vi "Autonomous Independent.vi"() -> ()   [LabVIEW 2020]
doc: "This VI is called when autonomous begins, and will automatically be terminated when autonomous ends. You can carry out timed or sensor driven robot movement independently without needing to return to the caller."
uses:
  <vilib>/Rock Robotics/WPI/Solenoid/WPI_SolenoidValue.ctl
  <vilib>/Rock Robotics/WPI/Utilities/WPI_GetSetVariantRefNum.vi
  <vilib>/Rock Robotics/Network Tables/NT Read String.vi
  <vilib>/Rock Robotics/Network Tables/NT Write Numeric Array.vi
  <vilib>/Rock Robotics/WPI/Solenoid/WPI_SolenoidSetEnum.vi
  <vilib>/Rock Robotics/WPI/RobotDrive/WPI_RobotDriveArcadeDrive_Standard(NoSaturation).vi
  Robot Global Data.vi
panel:
  out "Current Movement, for debugging":T1 {"Y Joystick Value" scale=1.0..-1.0; "X Joystick Value" scale=-1.0..1.0}
  in  "Array of robot movements":T2(array[cluster])=[{"X Joystick Value"=0.39393939393939403, "Y Joystick Value"=0.0, "Delay (sec)"=1.0, "Movement Name"="turn"}, {"X Joystick Value"=-0.3737373737373737, "Y Joystick Value"=0.0, "Delay (sec)"=1.0, "Movement Name"="turn back"}] {"Y Joystick Value" scale=1.0..-1.0; "X Joystick Value" scale=-1.0..1.0}
  # "Be sure to right-click and choose Data Operations>>Make Current Value default if you want to save the array values with the VI"
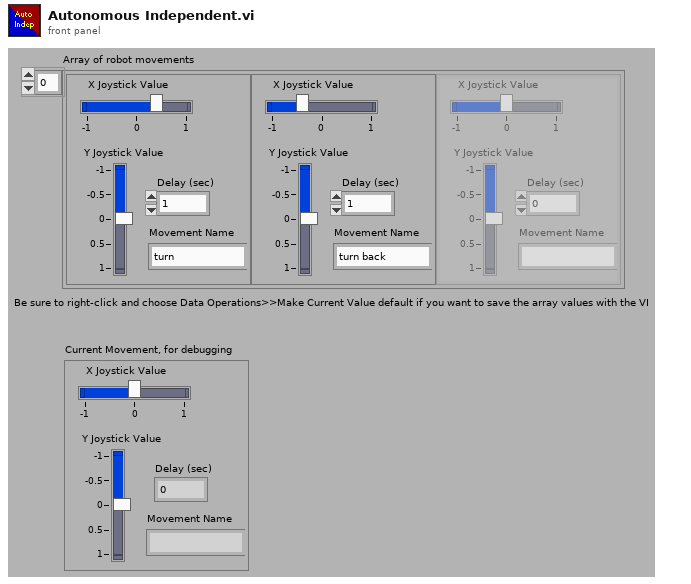
[diagram p1: front panel]
types:
  T1 = cluster{"X Joystick Value":dbl, "Y Joystick Value":dbl, "Delay (sec)":dbl, "Movement Name":string}
  T2 = cluster{"X Joystick Value":dbl, "Y Joystick Value":dbl, "Delay (sec)":dbl, "Movement Name":string}[]
  T3 = typedef "WPI_JoystickDevRef.ctl" = cluster{"Device":T4}
  T4 = typedef "WPI_JoystickDeviceEnum.ctl" = enum16{"USB 0", "USB 1", "USB 2", "USB 3", "USB 4", "USB 5"}
  T5 = typedef "WPI_SolenoidValue.ctl" = enum16{"Off", "On", "Forward", "Reverse"}
  T6 = typedef "WPI_MotorControlDeviceRef.ctl" = cluster{"DeviceStatus":errorcluster, "Type":T7, "PWM":cluster{"PWM Channel":T8, "DeadBand":T9}, "CAN":cluster{"Device Number":u8, "SetOutput VI Ref":variant, "GetOutput VI Ref":variant, "Enable VI Ref":variant, "Disable VI Ref":variant, "Data":variant}, "Invert":bool, "DIO PWM":cluster{"PWM \"Enable\" Channel":T8, "DIOChannel":T10, "PWM Rate":dbl}}
  T7 = typedef "WPI_MotorControlType.ctl" = enum16{"PWM", "CAN", "DIO PWM"}
  T8 = typedef "FPGA_DIOPWMChannel.ctl" = enum8{"PWM 0", "PWM 1", "PWM 2", "PWM 3", "PWM 4", "PWM 5", "PWM 6", "PWM 7", "PWM 8", "PWM 9", "PWM MXP 0", "PWM MXP 1", "PWM MXP 2", "PWM MXP 3", "PWM MXP 4", "PWM MXP 5", "PWM MXP 6", "PWM MXP 7", "PWM MXP 8", "PWM MXP 9", "Invalid"}
  T9 = typedef "WPI_PWMDeadband.ctl" = cluster{"Name":string, "maxPositivePwm":i32, "minPositivePwm":i32, "centerPwm":i32, "maxNegativePwm":i32, "minNegativePwm":i32, "angularRange":u16}
  T10 = typedef "FPGA_DIOChannel.ctl" = enum8{"DIO 0", "DIO 1", "DIO 2", "DIO 3", "DIO 4", "DIO 5", "DIO 6", "DIO 7", "DIO 8", "DIO 9", "DIO MXP 0", "DIO MXP 1", "DIO MXP 2", "DIO MXP 3", "DIO MXP 4", "DIO MXP 5", "DIO MXP 6", "DIO MXP 7", "DIO MXP 8", "DIO MXP 9", "DIO MXP 10", "DIO MXP 11", "DIO MXP 12", "DIO MXP 13", "DIO MXP 14", "DIO MXP 15", "SPI Port CS1", "SPI Port CS2", "SPI Port CS3", "SPI Port MISO", "SPI Port MOSI", "Invalid"}
  T11 = typedef "WPI_SolenoidDevRef.ctl" = cluster{"DevStatus":errorcluster, "Pneumatics Control Module":u8, "Forward Solenoid Channel":T12, "Reverse Solenoid Channel":T12}
  T12 = typedef "WPI_SolenoidChannel.ctl" = enum8{"Solenoid 0", "Solenoid 1", "Solenoid 2", "Solenoid 3", "Solenoid 4", "Solenoid 5", "Solenoid 6", "Solenoid 7", "Solenoid 8", "Solenoid 9", "Solenoid 10", "Solenoid 11", "Solenoid 12", "Solenoid 13", "Solenoid 14", "Solenoid 15", "Invalid"}
  T13 = typedef "WPI_RobotDriveDevRef.ctl" = cluster{"DevStatus":errorcluster, "Motors[]":T6[], "Square Inputs":bool, "Max Output":dbl}
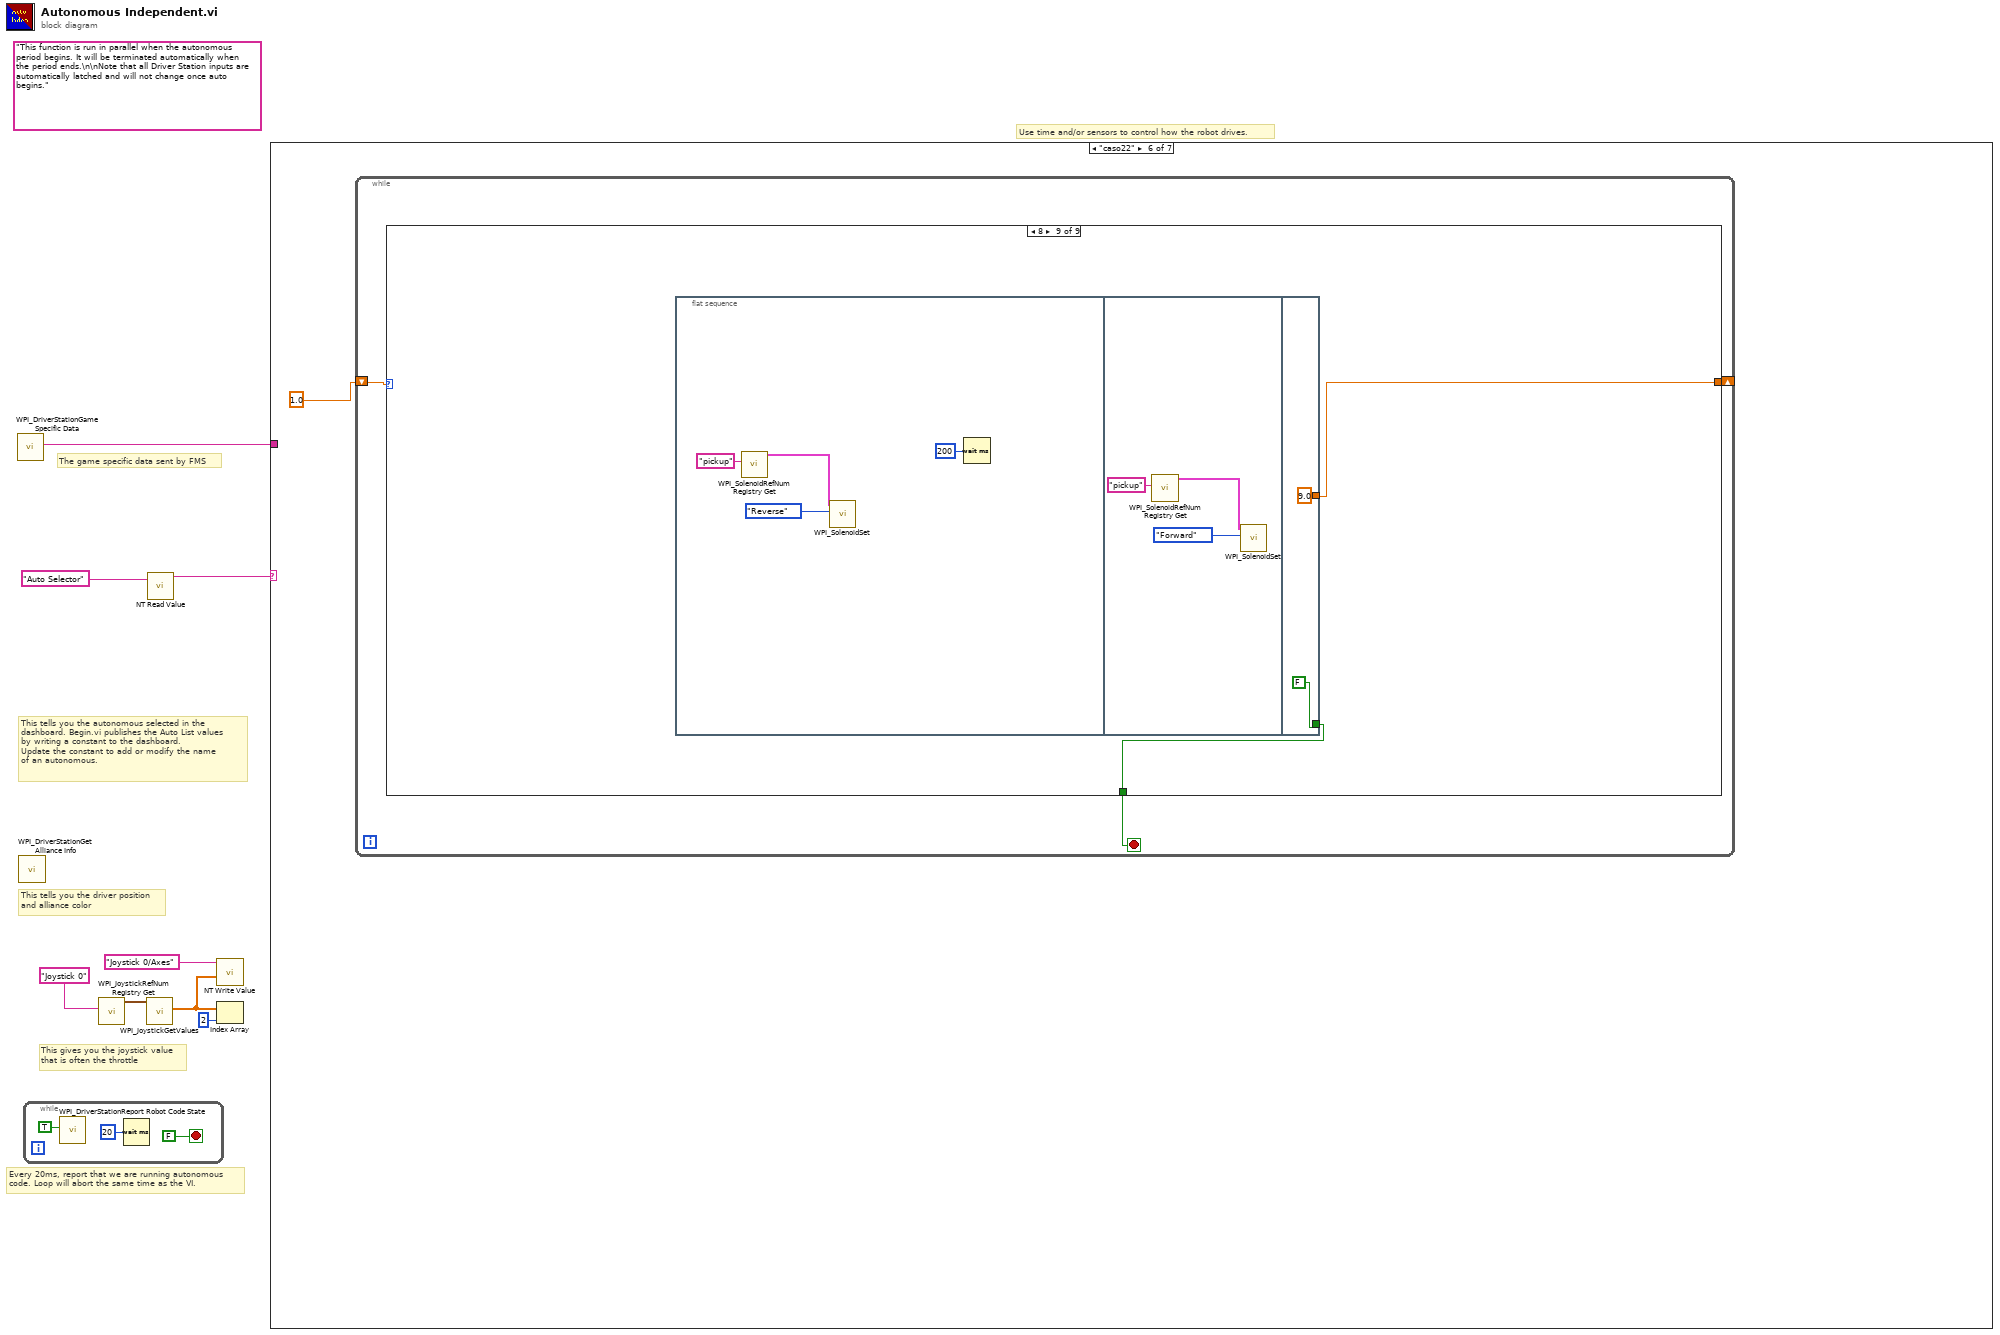
[diagram p0: block diagram]
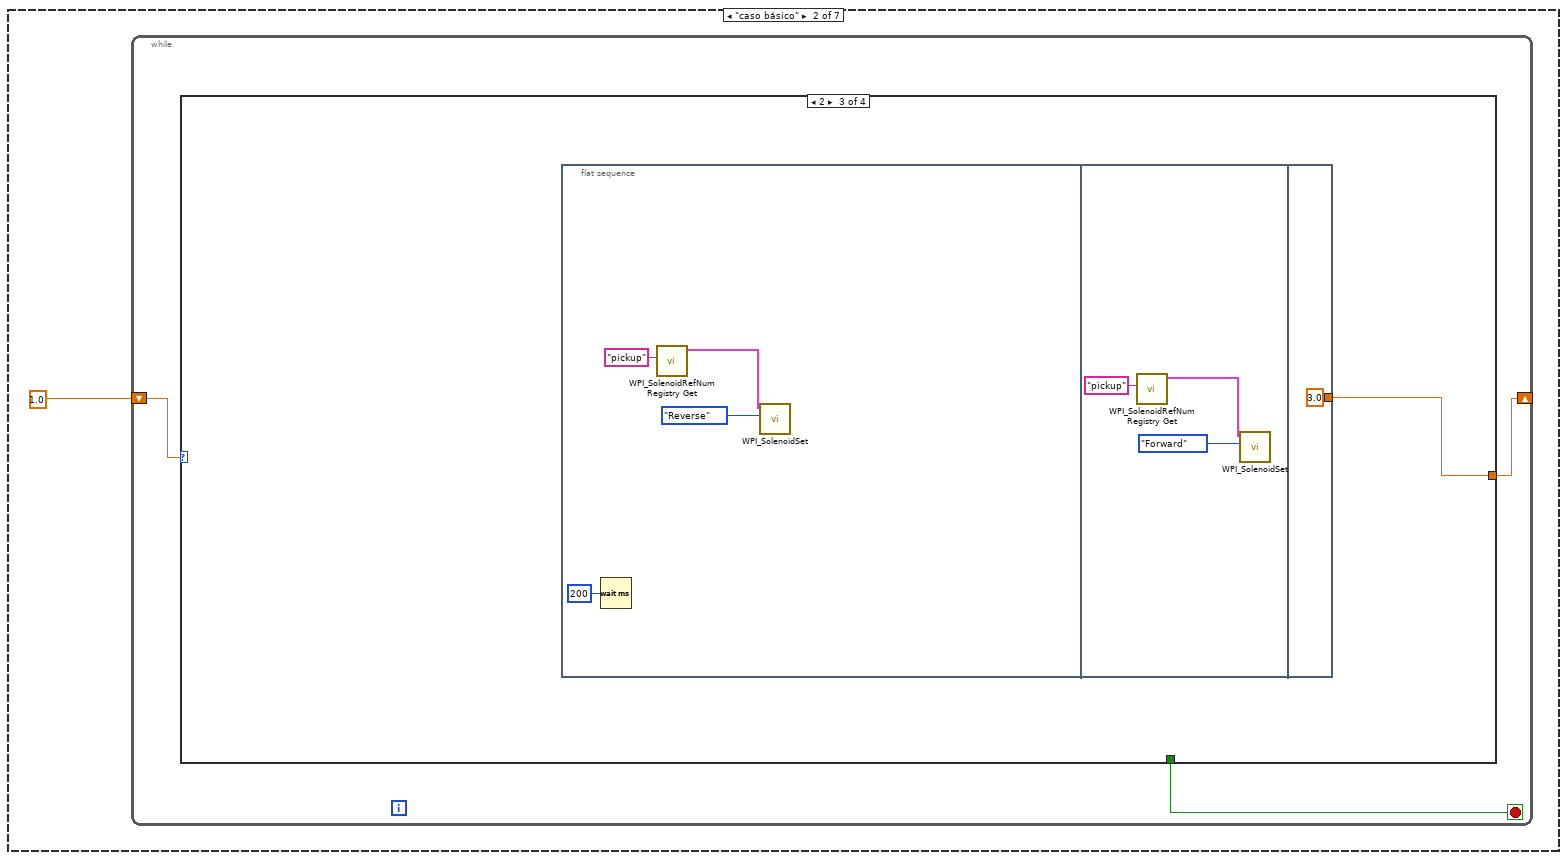
[diagram p3: hidden frame]
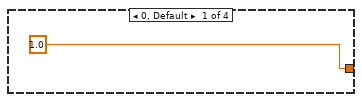
[diagram p4: hidden frame]
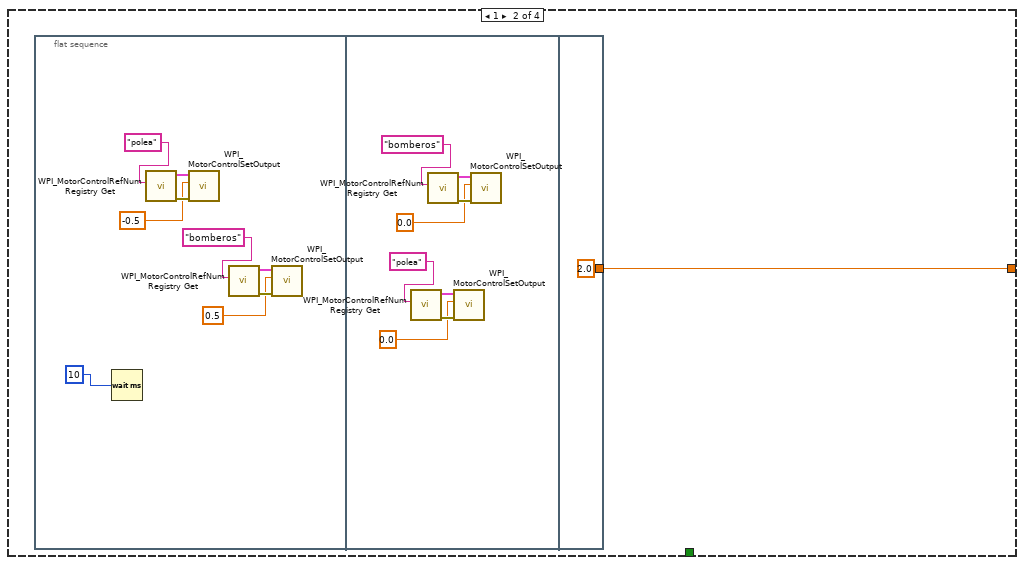
[diagram p5: hidden frame]
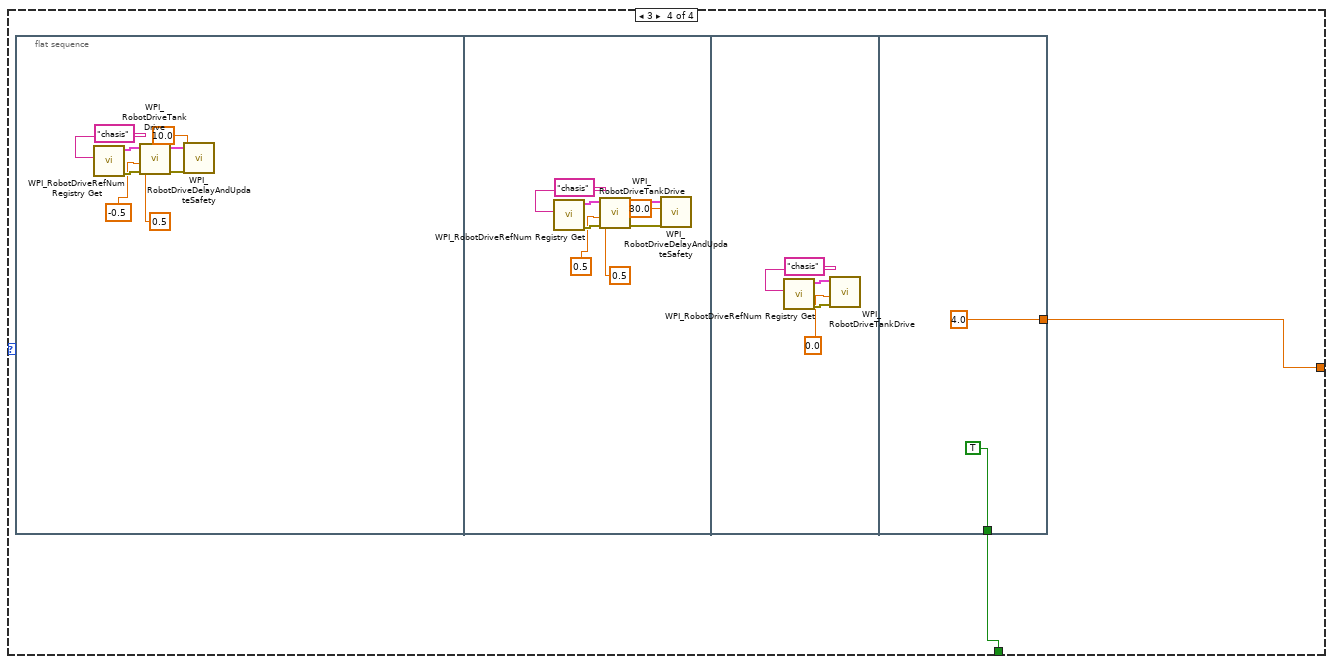
[diagram p6: hidden frame]
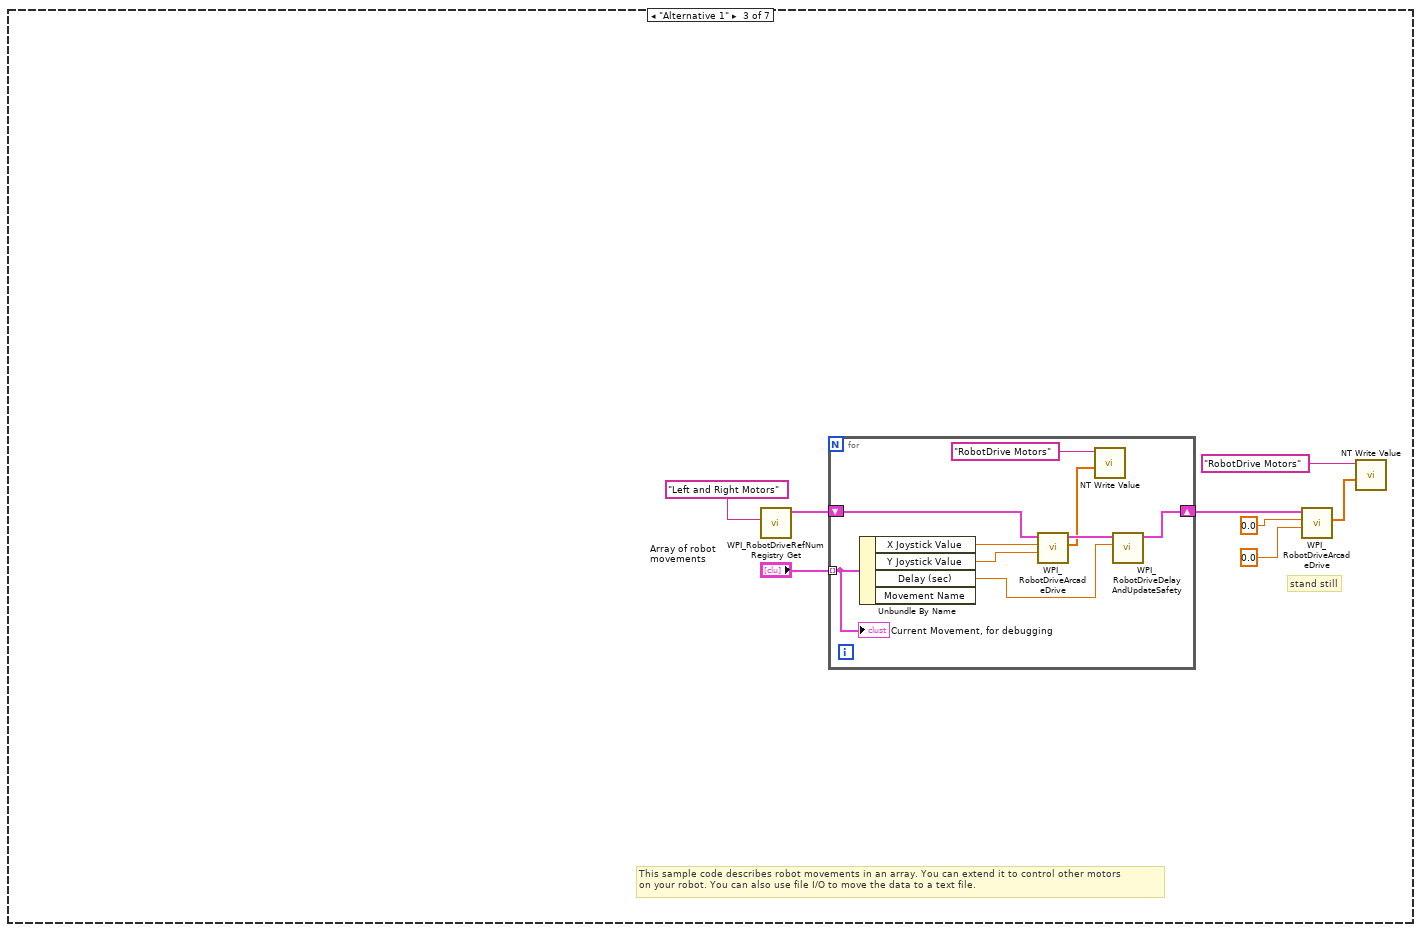
[diagram p7: hidden frame]
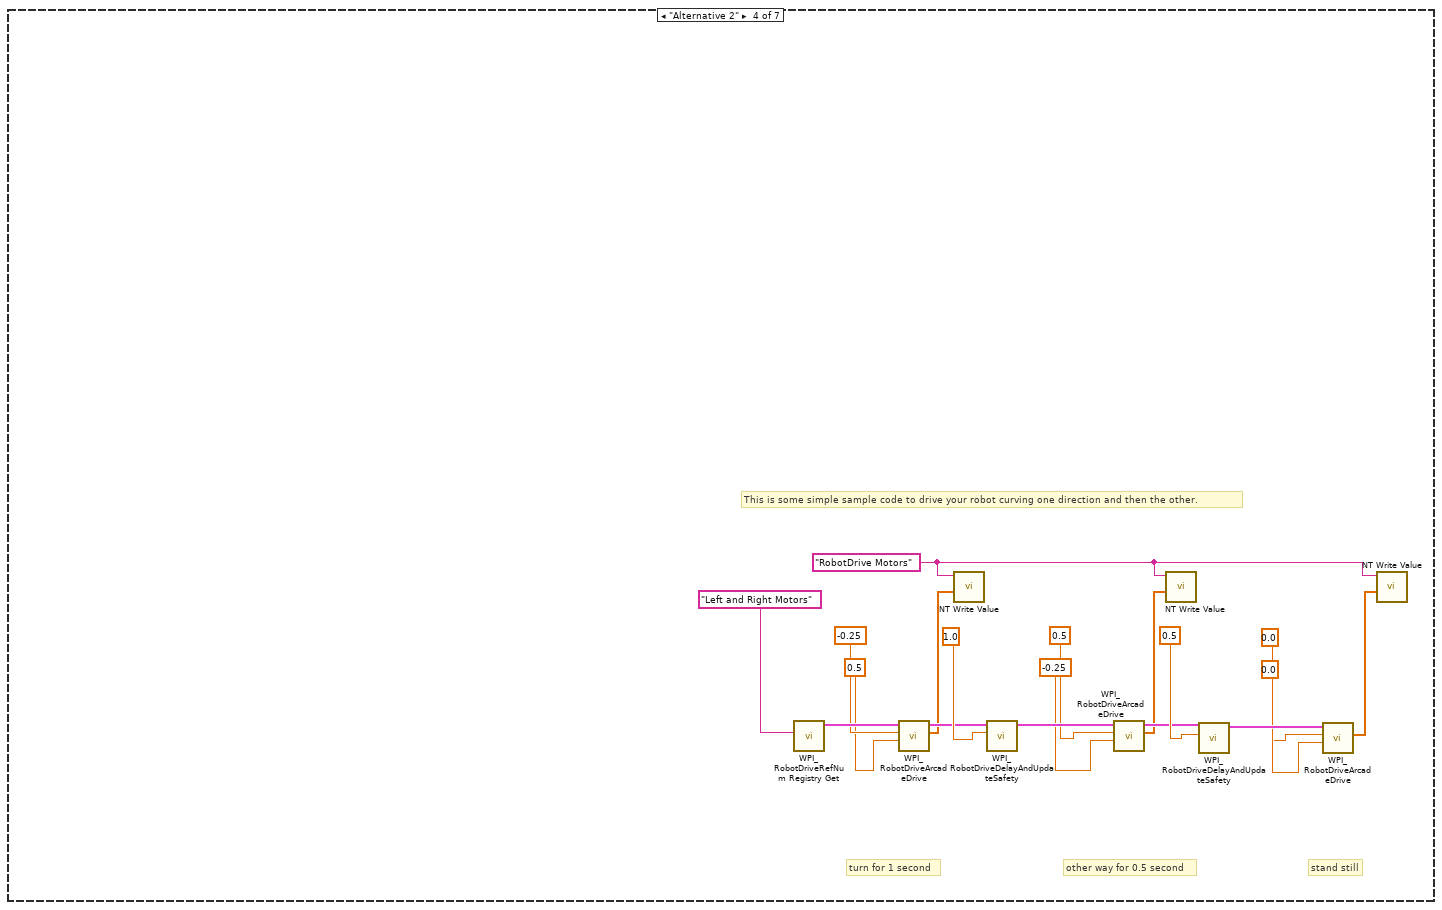
[diagram p8: hidden frame]
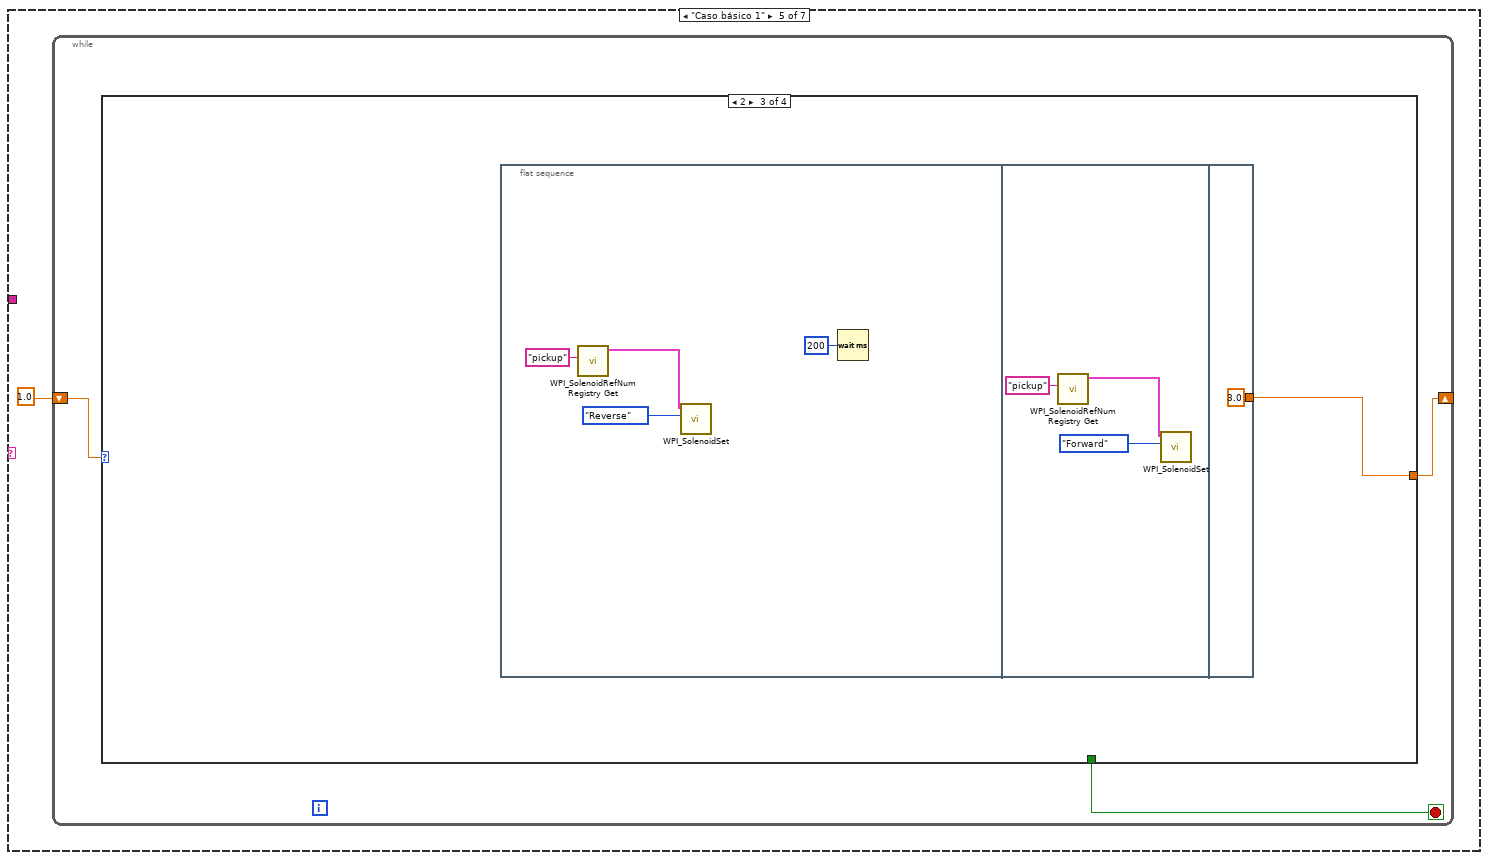
[diagram p9: hidden frame]
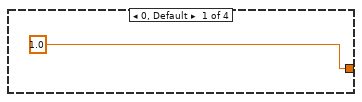
[diagram p10: hidden frame]
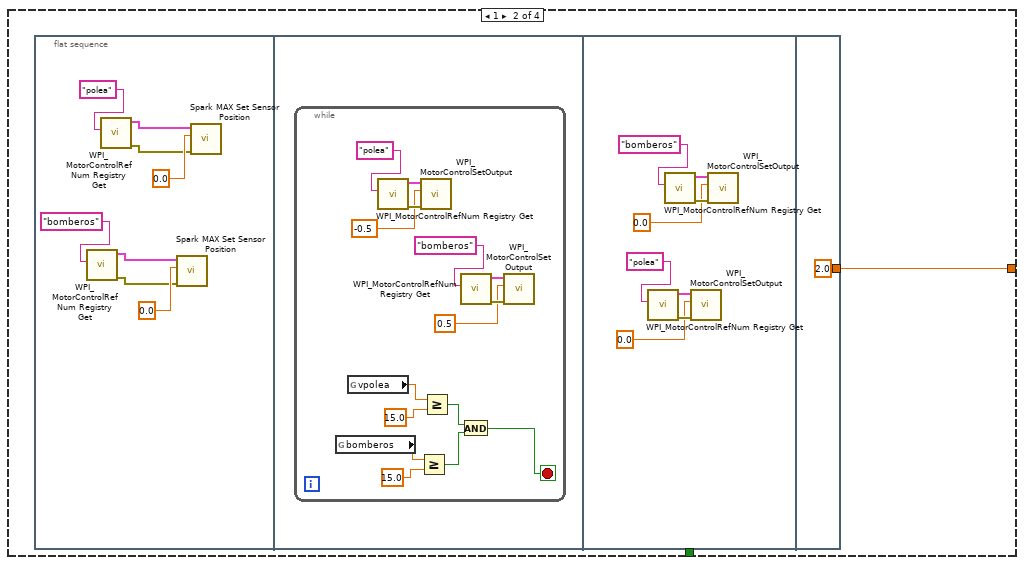
[diagram p11: hidden frame]
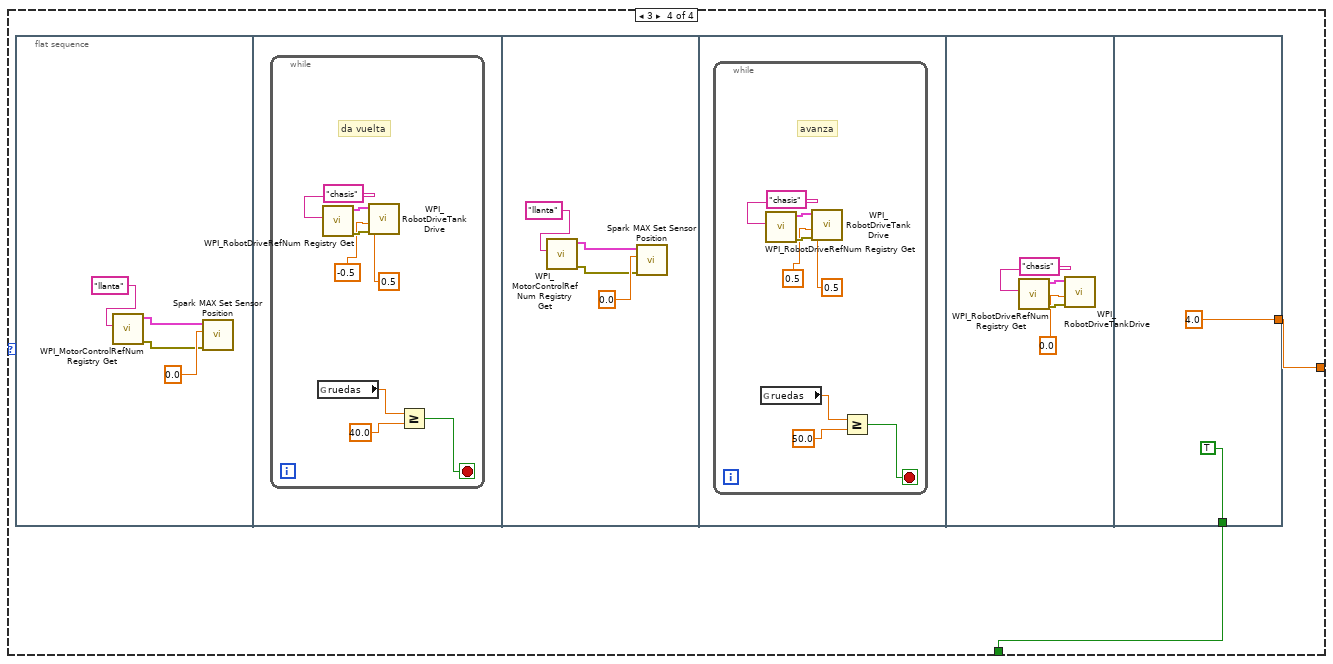
[diagram p12: hidden frame]
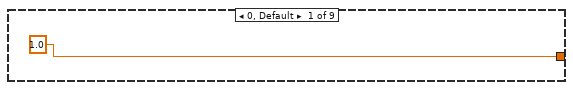
[diagram p13: hidden frame]
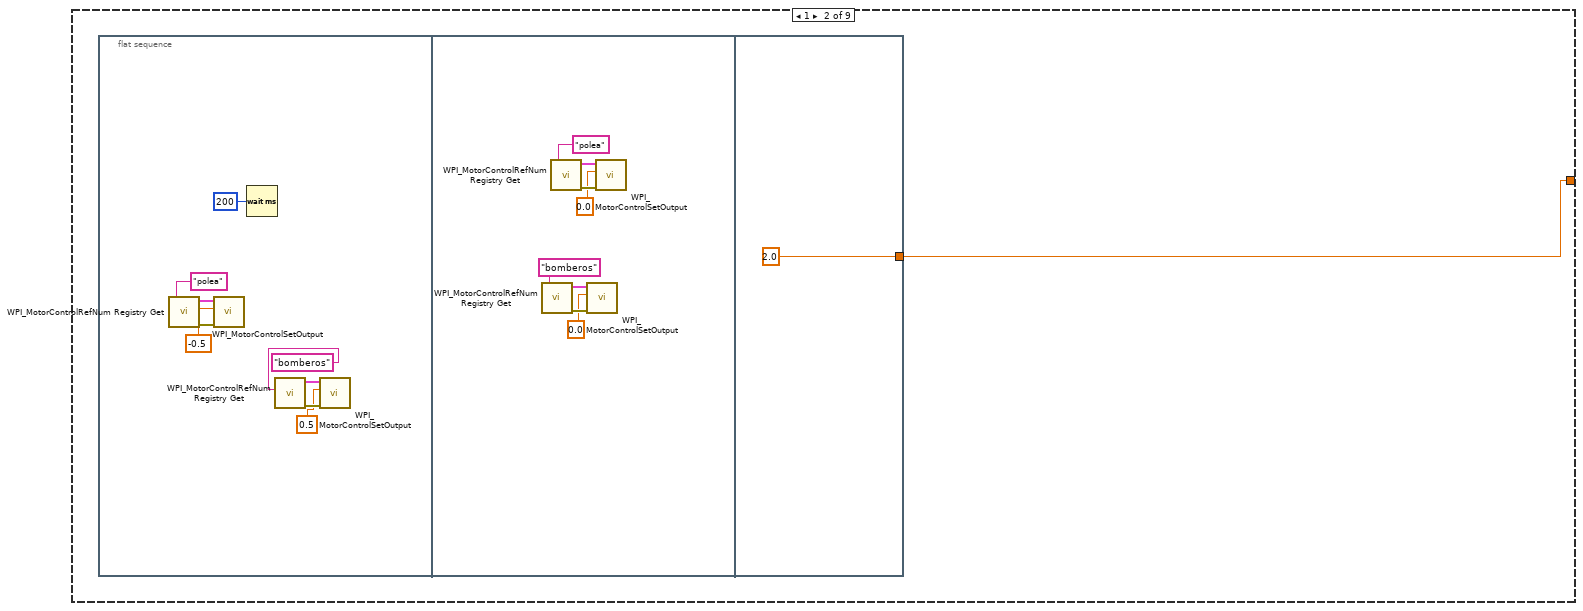
[diagram p14: hidden frame]
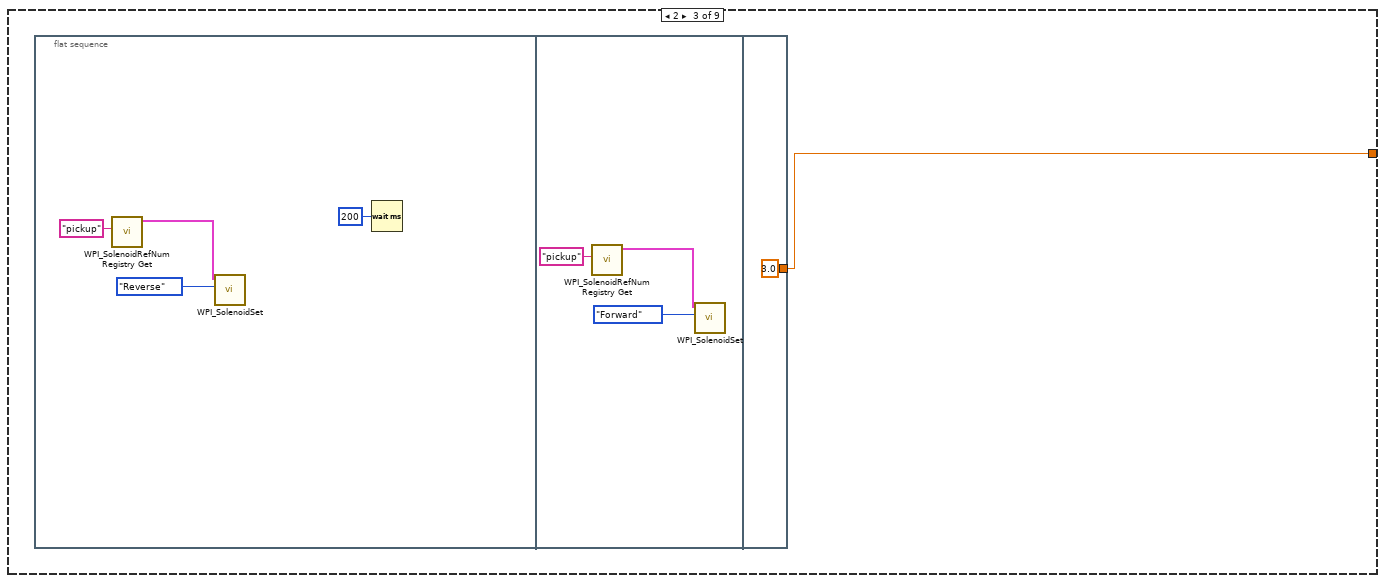
[diagram p15: hidden frame]
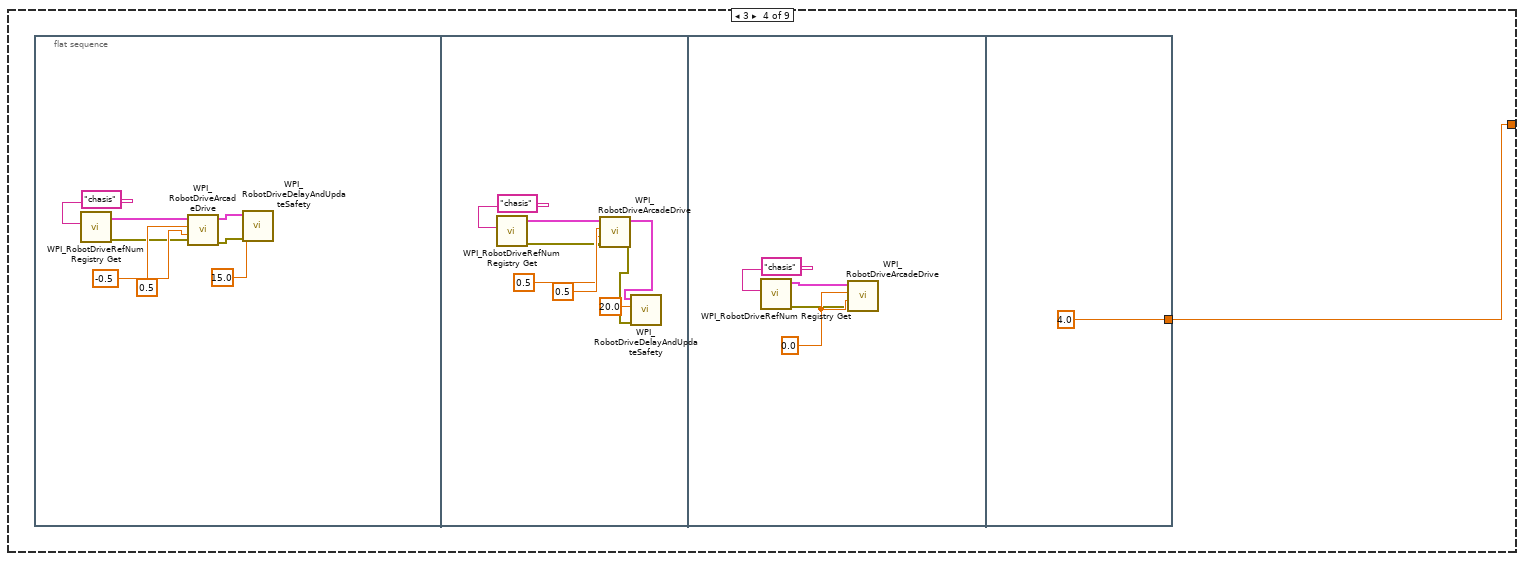
[diagram p16: hidden frame]
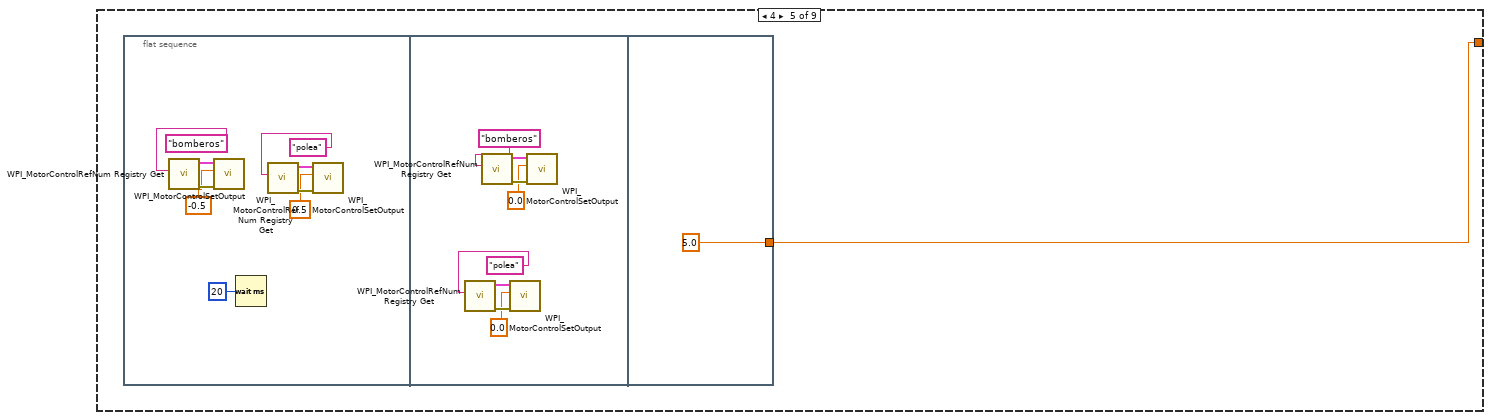
[diagram p17: hidden frame]
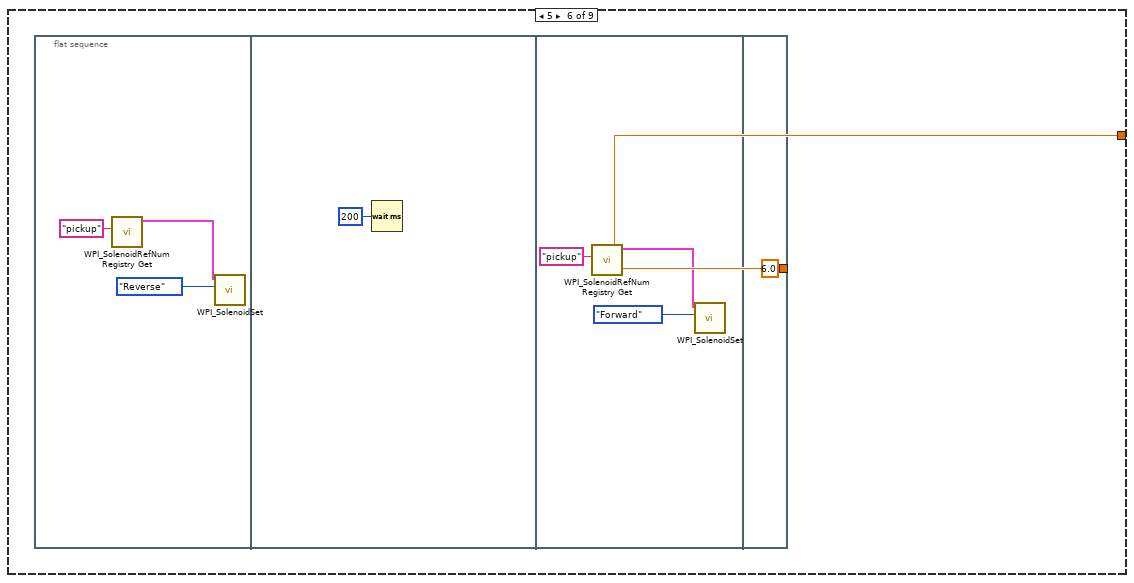
[diagram p18: hidden frame]
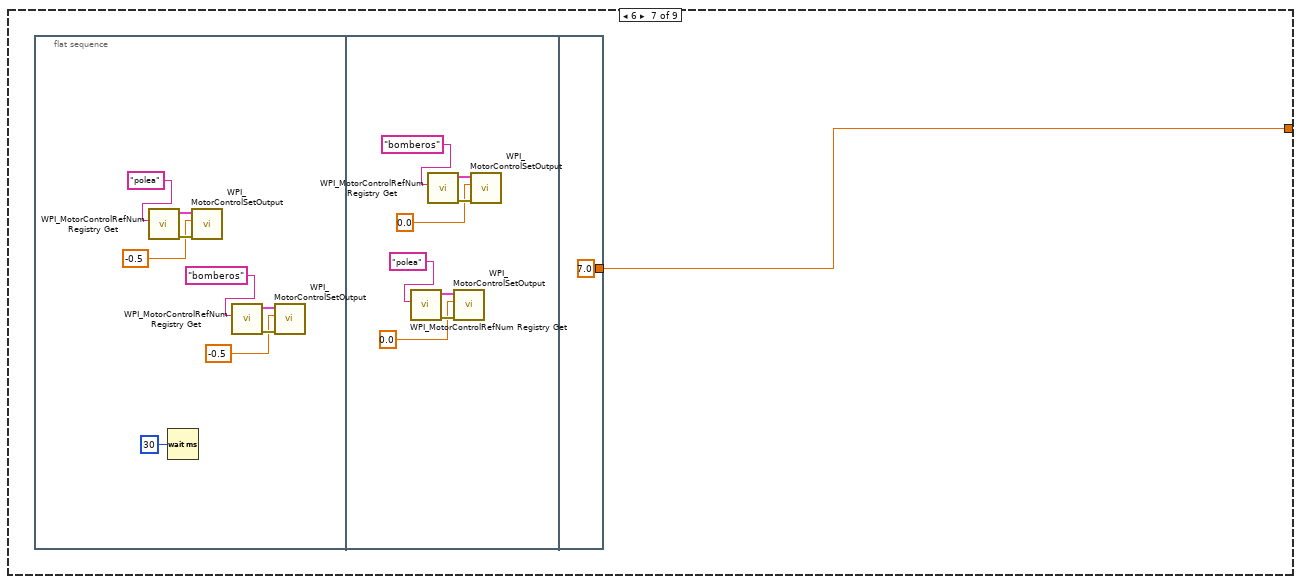
[diagram p19: hidden frame]
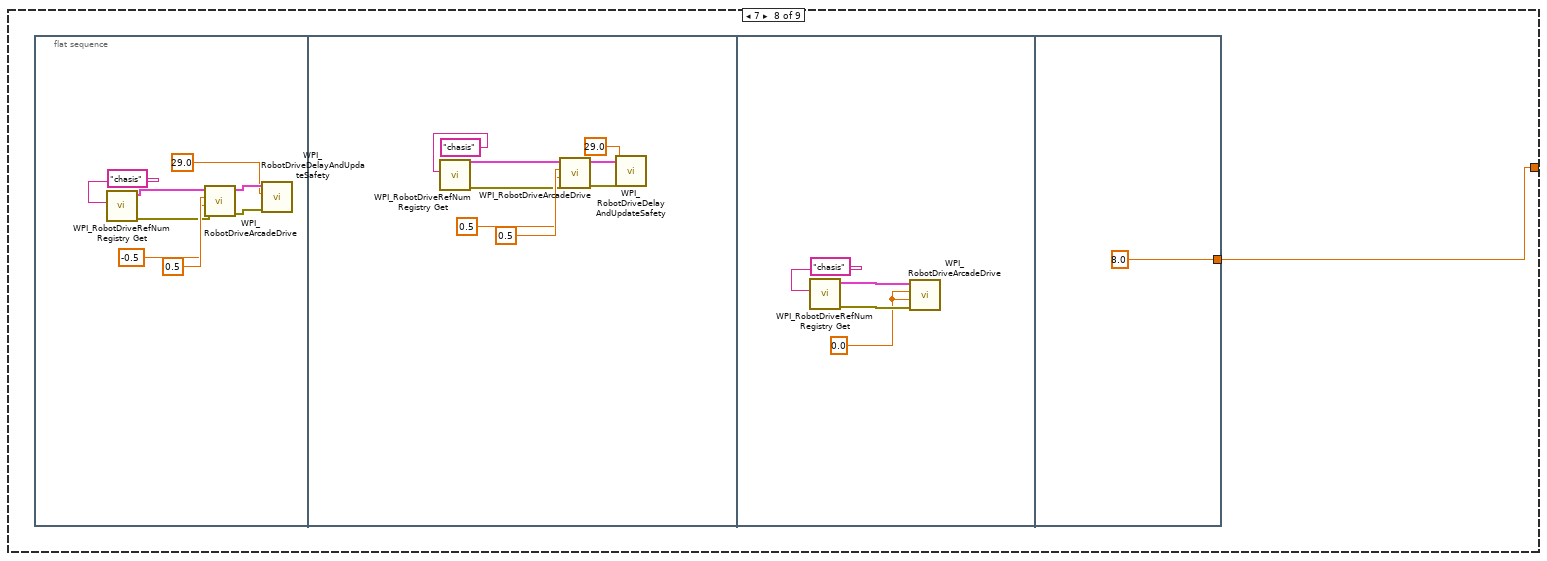
[diagram p20: hidden frame]
diagram:
  (unwired) "This function is run in parallel when the autonomous period begins. It will be terminated automatically when the period ends.\n\nNote that all Driver Station inputs are automatically latched and will not change once auto begins."
  # "The game specific data sent by FMS"
  # "This tells you the autonomous selected in the \ndashboard. Begin.vi publishes the Auto List values\nby writing a constant to the dashboard.\nUpdate the constant to add or modify the name\nof an autonomous."
  # "Every 20ms, report that we are running autonomous\ncode. Loop will abort the same time as the VI."
  # "This gives you the joystick value\nthat is often the throttle"
  # "Use time and/or sensors to control how the robot drives."
  # "This tells you the driver position\nand alliance color"
  n1 = call <vilib>:"WPI_DriverStationGame Specific Data.vi"() -> ("Game Specific Data"=w1:string)  [unwired: 11 in]
  n2 = call <vilib>:"WPI_DriverStationGet Alliance Info.vi"() -> ()  [unwired: 12 out]
  n3 = while {
    stop <- FALSE stop-if-true
    n4 = call <vilib>:"WPI_DriverStationReport Robot Code State.vi"("Autonomous"=TRUE) -> ()  [unwired: 10 in, 1 out]
    n5 = Wait (ms)(milliseconds to wait=u32 20) -> ()  [unwired: 1 out]
  }
  n6 = call <vilib>:"WPI_JoystickRefNum Registry Get.vi"("refnum name"="Joystick 0") -> ("JoystickDevRef"=w7:T3)  [unwired: 1 in, 9 out]
  n7 = call <vilib>:"WPI_JoystickGetValues.vi"("JoystickDevRef"=w7) -> ("Axes"=w3:dbl[])  [unwired: 6 in, 4 out]
  n8 = call-poly <vilib>:"NT Read Value.vi"("Name"="Auto Selector") -> ("String"=w4:string)  [unwired: 9 in, 1 out]
  n9 = call-poly <vilib>:"NT Write Value.vi"("Numeric Array"=w3, "Name"="Joystick 0/Axes") -> ()  [unwired: 9 in, 1 out]
  n10 = Index Array(array=w3, index=2) -> ()  [unwired: 1 out]
  n11 = case shown="\"caso22\"" w4 {
    tunnel: w1 -> [_ _ _ _ _ _ _]
    frame Default {
      # "You can put your main auto here, or you can right-click on the case and make any\nother frame be the default case."
      # "This is the frame that will execute if no selection is made, or if it is not recognized"
    }
    frame "caso básico" {
      n12 = while {
        shift-right: [w15] -> _
        shift-left: 1.0 -> [w13]
        stop <- w14 stop-if-true
        n13 = case shown="2" w13 {
          tunnel: [1.0 w17 w36 w46] -> w15
          tunnel: [_ _ _ w45] -> w14
          frame 0, Default {
          }
          frame 1 {
            n14 = flat-sequence {
              tunnel: [2.0] -> w17
              frame #0 {
                n15 = Wait (ms)(milliseconds to wait=u32 10 ("millisecond timer value")) -> ()  [unwired: 1 out]
                n16 = call <vilib>:"WPI_MotorControlRefNum Registry Get.vi"("refnum name"="polea") -> ("error out"=w26:errorcluster, "MotorControlDevRef"=w25:T6)  [unwired: 9 in]
                n17 = call <vilib>:"WPI_MotorControlSetOutput.vi"("error in (no error)"=w26, "Output"=-0.5, "MotorControlDevRef"=w25) -> ()  [unwired: 6 in, 3 out]
                n18 = call <vilib>:"WPI_MotorControlRefNum Registry Get.vi"("refnum name"="bomberos") -> ("error out"=w22:errorcluster, "MotorControlDevRef"=w21:T6)  [unwired: 9 in]
                n19 = call <vilib>:"WPI_MotorControlSetOutput.vi"("error in (no error)"=w22, "Output"=0.5, "MotorControlDevRef"=w21) -> ()  [unwired: 6 in, 3 out]
              }
              frame #1 {
                n20 = call <vilib>:"WPI_MotorControlRefNum Registry Get.vi"("refnum name"="polea") -> ("error out"=w33:errorcluster, "MotorControlDevRef"=w34:T6)  [unwired: 9 in]
                n21 = call <vilib>:"WPI_MotorControlRefNum Registry Get.vi"("refnum name"="bomberos") -> ("error out"=w29:errorcluster, "MotorControlDevRef"=w30:T6)  [unwired: 9 in]
                n22 = call <vilib>:"WPI_MotorControlSetOutput.vi"("error in (no error)"=w33, "Output"=0.0, "MotorControlDevRef"=w34) -> ()  [unwired: 6 in, 3 out]
                n23 = call <vilib>:"WPI_MotorControlSetOutput.vi"("error in (no error)"=w29, "Output"=0.0, "MotorControlDevRef"=w30) -> ()  [unwired: 6 in, 3 out]
              }
              frame #2 {
              }
            }
          }
          frame 2 {
            n24 = flat-sequence {
              tunnel: [3.0] -> w36
              frame #0 {
                n25 = Wait (ms)(milliseconds to wait=u32 200) -> ()  [unwired: 1 out]
                n26 = call <vilib>:"WPI_SolenoidRefNum Registry Get.vi"("refnum name"="pickup") -> ("SolenoidDevRef"=w40:T11)  [unwired: 9 in, 1 out]
                n27 = call-poly <vilib>:"WPI_SolenoidSet.vi"("Value"=WPI_SolenoidValue."Reverse", "SolenoidDevRef"=w40) -> ()  [unwired: 8 in, 2 out]
              }
              frame #1 {
                n28 = call <vilib>:"WPI_SolenoidRefNum Registry Get.vi"("refnum name"="pickup") -> ("SolenoidDevRef"=w43:T11)  [unwired: 9 in, 1 out]
                n29 = call-poly <vilib>:"WPI_SolenoidSet.vi"("Value"=WPI_SolenoidValue."Forward", "SolenoidDevRef"=w43) -> ()  [unwired: 8 in, 2 out]
              }
              frame #2 {
              }
            }
          }
          frame 3 {
            n30 = flat-sequence {
              tunnel: [4.0] -> w46
              tunnel: [TRUE] -> w45
              frame #0 {
                n31 = call <vilib>:"WPI_RobotDriveRefNum Registry Get.vi"("refnum name"="chasis") -> ("error out"=w54:errorcluster, "RobotDriveDevRef"=w53:T13)  [unwired: 9 in]
                n32 = call <vilib>:"WPI_RobotDriveTankDrive.vi"("error in (no error)"=w54, "Right axis value"=-0.5 ("Motor Output"), "Left axis value"=0.5 ("Motor Output"), "RobotDriveDevRef"=w53) -> ("error out"=w49:errorcluster, "RobotDriveDevRef"=w48:T13)  [unwired: 5 in, 1 out]
                n33 = call <vilib>:"WPI_RobotDriveDelayAndUpdateSafety.vi"("error in (no error)"=w49, "Delay (s)"=10.0, "RobotDriveDevRef"=w48) -> ()  [unwired: 7 in, 2 out]
              }
              frame #1 {
                n34 = call <vilib>:"WPI_RobotDriveRefNum Registry Get.vi"("refnum name"="chasis") -> ("error out"=w62:errorcluster, "RobotDriveDevRef"=w61:T13)  [unwired: 9 in]
                n35 = call <vilib>:"WPI_RobotDriveTankDrive.vi"("error in (no error)"=w62, "Right axis value"=0.5 ("Motor Output"), "Left axis value"=0.5 ("Motor Output"), "RobotDriveDevRef"=w61) -> ("error out"=w56:errorcluster, "RobotDriveDevRef"=w57:T13)  [unwired: 5 in, 1 out]
                n36 = call <vilib>:"WPI_RobotDriveDelayAndUpdateSafety.vi"("error in (no error)"=w56, "Delay (s)"=30.0, "RobotDriveDevRef"=w57) -> ()  [unwired: 7 in, 2 out]
              }
              frame #2 {
                n37 = call <vilib>:"WPI_RobotDriveRefNum Registry Get.vi"("refnum name"="chasis") -> ("error out"=w66:errorcluster, "RobotDriveDevRef"=w65:T13)  [unwired: 9 in]
                n38 = call <vilib>:"WPI_RobotDriveTankDrive.vi"("error in (no error)"=w66, "Right axis value"=0.0 ("Motor Output"), "RobotDriveDevRef"=w65) -> ()  [unwired: 6 in, 3 out]
              }
              frame #3 {
              }
            }
          }
        }
      }
    }
    frame "Alternative 1" {
      # "stand still"
      # "This sample code describes robot movements in an array. You can extend it to control other motors\non your robot. You can also use file I/O to move the data to a text file."
      n39 = call <vilib>:"WPI_RobotDriveRefNum Registry Get.vi"("refnum name"="Left and Right Motors") -> ("RobotDriveDevRef"=w75:T13)  [unwired: 1 in, 9 out]
      n40 = for {
        shift-right: [w83] -> w70
        shift-left: w75 -> [w84]
        tunnel: "Array of robot movements" -> [w79] mode=indexing
        n41 = Unbundle By Name(w79) -> ("X Joystick Value"=w82:dbl, "Y Joystick Value"=w81:dbl, "Delay (sec)"=w80:dbl)  [unwired: 1 out]
        n42 = call-poly <vilib>:"WPI_RobotDriveArcadeDrive.vi"("Y axis value"=w81, "X axis value"=w82, "RobotDriveDevRef"=w84) -> ("Motor Values"=w77:dbl[], "RobotDriveDevRef"=w85:T13)  [unwired: 1 in, 6 out]
        n43 = call-poly <vilib>:"NT Write Value.vi"("Numeric Array"=w77, "Name"="RobotDrive Motors") -> ()  [unwired: 9 in, 1 out]
        n44 = call <vilib>:"WPI_RobotDriveDelayAndUpdateSafety.vi"("Delay (s)"=w80, "RobotDriveDevRef"=w85) -> ("RobotDriveDevRef 2"=w83:T13)  [unwired: 8 in, 1 out]
        "Current Movement, for debugging" <- w79
      }
      n45 = call-poly <vilib>:"WPI_RobotDriveArcadeDrive.vi"("Y axis value"=0.0 ("X axis value"), "X axis value"=0.0, "RobotDriveDevRef"=w70) -> ("Motor Values"=w73:dbl[])  [unwired: 1 in, 7 out]
      n46 = call-poly <vilib>:"NT Write Value.vi"("Numeric Array"=w73, "Name"="RobotDrive Motors") -> ()  [unwired: 9 in, 1 out]
    }
    frame "Alternative 2" {
      w87 = "RobotDrive Motors" ("Name")
      # "This is some simple sample code to drive your robot curving one direction and then the other."
      # "stand still"
      # "other way for 0.5 second"
      # "turn for 1 second"
      n47 = call <vilib>:"WPI_RobotDriveRefNum Registry Get.vi"("refnum name"="Left and Right Motors") -> ("RobotDriveDevRef"=w103:T13)  [unwired: 1 in, 9 out]
      n48 = call-poly <vilib>:"WPI_RobotDriveArcadeDrive.vi"("Y axis value"=0.5 ("X axis value"), "X axis value"=-0.25, "RobotDriveDevRef"=w103) -> ("Motor Values"=w86:dbl[], "RobotDriveDevRef"=w96:T13)  [unwired: 1 in, 6 out]
      n49 = call-poly <vilib>:"NT Write Value.vi"("Numeric Array"=w86, "Name"=w87) -> ()  [unwired: 9 in, 1 out]
      n50 = call <vilib>:"WPI_RobotDriveDelayAndUpdateSafety.vi"("Delay (s)"=1.0, "RobotDriveDevRef"=w96) -> ("RobotDriveDevRef 2"=w97:T13)  [unwired: 8 in, 1 out]
      n51 = call-poly <vilib>:"WPI_RobotDriveArcadeDrive.vi"("Y axis value"=-0.25 ("X axis value"), "X axis value"=0.5, "RobotDriveDevRef"=w97) -> ("Motor Values"=w88:dbl[], "RobotDriveDevRef"=w98:T13)  [unwired: 1 in, 6 out]
      n52 = call-poly <vilib>:"NT Write Value.vi"("Numeric Array"=w88, "Name"=w87) -> ()  [unwired: 9 in, 1 out]
      n53 = call <vilib>:"WPI_RobotDriveDelayAndUpdateSafety.vi"("Delay (s)"=0.5, "RobotDriveDevRef"=w98) -> ("RobotDriveDevRef 2"=w99:T13)  [unwired: 8 in, 1 out]
      n54 = call-poly <vilib>:"WPI_RobotDriveArcadeDrive.vi"("Y axis value"=0.0 ("X axis value"), "X axis value"=0.0, "RobotDriveDevRef"=w99) -> ("Motor Values"=w89:dbl[])  [unwired: 1 in, 7 out]
      n55 = call-poly <vilib>:"NT Write Value.vi"("Numeric Array"=w89, "Name"=w87) -> ()  [unwired: 9 in, 1 out]
    }
    frame "Caso básico 1" {
      n56 = while {
        shift-right: [w107] -> _
        shift-left: 1.0 -> [w105]
        stop <- w106 stop-if-true
        n57 = case shown="2" w105 {
          tunnel: [1.0 w109 w142 w152] -> w107
          tunnel: [_ _ _ w151] -> w106
          frame 0, Default {
          }
          frame 1 {
            n58 = flat-sequence {
              tunnel: [2.0] -> w109
              frame #0 {
                n59 = call <vilib>:"WPI_MotorControlRefNum Registry Get.vi"("refnum name"="bomberos") -> ("error out"=w110:errorcluster, "MotorControlDevRef"=w111:T6)  [unwired: 9 in]
                n60 = call <vilib>:"WPI_MotorControlRefNum Registry Get.vi"("refnum name"="polea") -> ("error out"=w114:errorcluster, "MotorControlDevRef"=w115:T6)  [unwired: 9 in]
                n61 = call <vilib>:"Spark MAX Set Sensor Position.vi"("error in"=w110, "Position"=0.0, "MotorControlDeviceRef"=w111) -> ()  [unwired: 7 in, 2 out]
                n62 = call <vilib>:"Spark MAX Set Sensor Position.vi"("error in"=w114, "Position"=0.0, "MotorControlDeviceRef"=w115) -> ()  [unwired: 7 in, 2 out]
              }
              frame #1 {
                n63 = while {
                  stop <- w121 stop-if-true
                  n64 = global read "Robot Global Data.vi" "bomberos"() -> (w120:dbl)
                  n65 = global read "Robot Global Data.vi" "vpolea"() -> (w128:dbl)
                  n66 = call <vilib>:"WPI_MotorControlRefNum Registry Get.vi"("refnum name"="polea") -> ("error out"=w132:errorcluster, "MotorControlDevRef"=w131:T6)  [unwired: 9 in]
                  n67 = Greater Or Equal?(x=w120, y=15.0) -> (x >= y?=w118:bool)
                  n68 = call <vilib>:"WPI_MotorControlSetOutput.vi"("error in (no error)"=w132, "Output"=-0.5, "MotorControlDevRef"=w131) -> ()  [unwired: 6 in, 3 out]
                  n69 = Greater Or Equal?(x=w128, y=15.0) -> (x >= y?=w122:bool)
                  n70 = call <vilib>:"WPI_MotorControlRefNum Registry Get.vi"("refnum name"="bomberos") -> ("error out"=w126:errorcluster, "MotorControlDevRef"=w125:T6)  [unwired: 9 in]
                  n71 = And(x=w122, y=w118) -> (x .and. y?=w121:bool)
                  n72 = call <vilib>:"WPI_MotorControlSetOutput.vi"("error in (no error)"=w126, "Output"=0.5, "MotorControlDevRef"=w125) -> ()  [unwired: 6 in, 3 out]
                }
              }
              frame #2 {
                n73 = call <vilib>:"WPI_MotorControlRefNum Registry Get.vi"("refnum name"="polea") -> ("error out"=w139:errorcluster, "MotorControlDevRef"=w140:T6)  [unwired: 9 in]
                n74 = call <vilib>:"WPI_MotorControlRefNum Registry Get.vi"("refnum name"="bomberos") -> ("error out"=w135:errorcluster, "MotorControlDevRef"=w136:T6)  [unwired: 9 in]
                n75 = call <vilib>:"WPI_MotorControlSetOutput.vi"("error in (no error)"=w139, "Output"=0.0, "MotorControlDevRef"=w140) -> ()  [unwired: 6 in, 3 out]
                n76 = call <vilib>:"WPI_MotorControlSetOutput.vi"("error in (no error)"=w135, "Output"=0.0, "MotorControlDevRef"=w136) -> ()  [unwired: 6 in, 3 out]
              }
              frame #3 {
              }
            }
          }
          frame 2 {
            n77 = flat-sequence {
              tunnel: [3.0] -> w142
              frame #0 {
                n78 = call <vilib>:"WPI_SolenoidRefNum Registry Get.vi"("refnum name"="pickup") -> ("SolenoidDevRef"=w145:T11)  [unwired: 9 in, 1 out]
                n79 = call-poly <vilib>:"WPI_SolenoidSet.vi"("Value"=WPI_SolenoidValue."Reverse", "SolenoidDevRef"=w145) -> ()  [unwired: 8 in, 2 out]
                n80 = Wait (ms)(milliseconds to wait=u32 200) -> ()  [unwired: 1 out]
              }
              frame #1 {
                n81 = call <vilib>:"WPI_SolenoidRefNum Registry Get.vi"("refnum name"="pickup") -> ("SolenoidDevRef"=w149:T11)  [unwired: 9 in, 1 out]
                n82 = call-poly <vilib>:"WPI_SolenoidSet.vi"("Value"=WPI_SolenoidValue."Forward", "SolenoidDevRef"=w149) -> ()  [unwired: 8 in, 2 out]
              }
              frame #2 {
              }
            }
          }
          frame 3 {
            n83 = flat-sequence {
              tunnel: [4.0] -> w152
              tunnel: [TRUE] -> w151
              frame #0 {
                n84 = call <vilib>:"WPI_MotorControlRefNum Registry Get.vi"("refnum name"="llanta") -> ("error out"=w153:errorcluster, "MotorControlDevRef"=w154:T6)  [unwired: 9 in]
                n85 = call <vilib>:"Spark MAX Set Sensor Position.vi"("error in"=w153, "Position"=0.0, "MotorControlDeviceRef"=w154) -> ()  [unwired: 7 in, 2 out]
              }
              frame #1 {
                n86 = while {
                  stop <- w157 stop-if-true
                  # "da vuelta"
                  n87 = global read "Robot Global Data.vi" "ruedas"() -> (w159:dbl)
                  n88 = call <vilib>:"WPI_RobotDriveRefNum Registry Get.vi"("refnum name"="chasis") -> ("error out"=w164:errorcluster, "RobotDriveDevRef"=w163:T13)  [unwired: 9 in]
                  n89 = call <vilib>:"WPI_RobotDriveTankDrive.vi"("error in (no error)"=w164, "Right axis value"=-0.5 ("Motor Output"), "Left axis value"=0.5 ("Motor Output"), "RobotDriveDevRef"=w163) -> ()  [unwired: 5 in, 3 out]
                  n90 = Greater Or Equal?(x=w159, y=40.0) -> (x >= y?=w157:bool)
                }
              }
              frame #2 {
                n91 = call <vilib>:"WPI_MotorControlRefNum Registry Get.vi"("refnum name"="llanta") -> ("error out"=w165:errorcluster, "MotorControlDevRef"=w166:T6)  [unwired: 9 in]
                n92 = call <vilib>:"Spark MAX Set Sensor Position.vi"("error in"=w165, "Position"=0.0, "MotorControlDeviceRef"=w166) -> ()  [unwired: 7 in, 2 out]
              }
              frame #3 {
                n93 = while {
                  stop <- w169 stop-if-true
                  # "avanza"
                  n94 = global read "Robot Global Data.vi" "ruedas"() -> (w171:dbl)
                  n95 = call <vilib>:"WPI_RobotDriveRefNum Registry Get.vi"("refnum name"="chasis") -> ("error out"=w176:errorcluster, "RobotDriveDevRef"=w175:T13)  [unwired: 9 in]
                  n96 = call <vilib>:"WPI_RobotDriveTankDrive.vi"("error in (no error)"=w176, "Right axis value"=0.5 ("Motor Output"), "Left axis value"=0.5 ("Motor Output"), "RobotDriveDevRef"=w175) -> ()  [unwired: 5 in, 3 out]
                  n97 = Greater Or Equal?(x=w171, y=50.0) -> (x >= y?=w169:bool)
                }
              }
              frame #4 {
                n98 = call <vilib>:"WPI_RobotDriveRefNum Registry Get.vi"("refnum name"="chasis") -> ("error out"=w180:errorcluster, "RobotDriveDevRef"=w179:T13)  [unwired: 9 in]
                n99 = call <vilib>:"WPI_RobotDriveTankDrive.vi"("error in (no error)"=w180, "Right axis value"=0.0 ("Motor Output"), "RobotDriveDevRef"=w179) -> ()  [unwired: 6 in, 3 out]
              }
              frame #5 {
              }
            }
          }
        }
      }
    }
    frame "caso22" {
      n100 = while {
        shift-right: [w185] -> _
        shift-left: 1.0 -> [w186]
        stop <- w184 stop-if-true
        n101 = case shown="8" w186 {
          tunnel: [1.0 w188 w207 w216 w238 w257 w266 w285 w308] -> w185
          tunnel: [_ _ _ _ _ _ _ _ w307] -> w184
          frame 0, Default {
          }
          frame 1 {
            n102 = flat-sequence {
              tunnel: [2.0] -> w188
              frame #0 {
                n103 = call <vilib>:"WPI_MotorControlRefNum Registry Get.vi"("refnum name"="polea") -> ("error out"=w196:errorcluster, "MotorControlDevRef"=w197:T6)  [unwired: 9 in]
                n104 = call <vilib>:"WPI_MotorControlSetOutput.vi"("error in (no error)"=w196, "Output"=-0.5 ("Motor Output"), "MotorControlDevRef"=w197) -> ()  [unwired: 6 in, 3 out]
                n105 = Wait (ms)(milliseconds to wait=u32 200) -> ()  [unwired: 1 out]
                n106 = call <vilib>:"WPI_MotorControlRefNum Registry Get.vi"("refnum name"="bomberos") -> ("error out"=w193:errorcluster, "MotorControlDevRef"=w192:T6)  [unwired: 9 in]
                n107 = call <vilib>:"WPI_MotorControlSetOutput.vi"("error in (no error)"=w193, "Output"=0.5 ("Motor Output"), "MotorControlDevRef"=w192) -> ()  [unwired: 6 in, 3 out]
              }
              frame #1 {
                n108 = call <vilib>:"WPI_MotorControlRefNum Registry Get.vi"("refnum name"="bomberos") -> ("error out"=w200:errorcluster, "MotorControlDevRef"=w201:T6)  [unwired: 9 in]
                n109 = call <vilib>:"WPI_MotorControlRefNum Registry Get.vi"("refnum name"="polea") -> ("error out"=w204:errorcluster, "MotorControlDevRef"=w205:T6)  [unwired: 9 in]
                n110 = call <vilib>:"WPI_MotorControlSetOutput.vi"("error in (no error)"=w200, "Output"=0.0 ("Motor Output"), "MotorControlDevRef"=w201) -> ()  [unwired: 6 in, 3 out]
                n111 = call <vilib>:"WPI_MotorControlSetOutput.vi"("error in (no error)"=w204, "Output"=0.0 ("Motor Output"), "MotorControlDevRef"=w205) -> ()  [unwired: 6 in, 3 out]
              }
              frame #2 {
              }
            }
          }
          frame 2 {
            n112 = flat-sequence {
              tunnel: [3.0] -> w207
              frame #0 {
                n113 = call <vilib>:"WPI_SolenoidRefNum Registry Get.vi"("refnum name"="pickup") -> ("SolenoidDevRef"=w210:T11)  [unwired: 9 in, 1 out]
                n114 = call-poly <vilib>:"WPI_SolenoidSet.vi"("Value"=WPI_SolenoidValue."Reverse", "SolenoidDevRef"=w210) -> ()  [unwired: 8 in, 2 out]
                n115 = Wait (ms)(milliseconds to wait=u32 200) -> ()  [unwired: 1 out]
              }
              frame #1 {
                n116 = call <vilib>:"WPI_SolenoidRefNum Registry Get.vi"("refnum name"="pickup") -> ("SolenoidDevRef"=w214:T11)  [unwired: 9 in, 1 out]
                n117 = call-poly <vilib>:"WPI_SolenoidSet.vi"("Value"=WPI_SolenoidValue."Forward", "SolenoidDevRef"=w214) -> ()  [unwired: 8 in, 2 out]
              }
              frame #2 {
              }
            }
          }
          frame 3 {
            n118 = flat-sequence {
              tunnel: [4.0] -> w216
              frame #0 {
                n119 = call <vilib>:"WPI_RobotDriveRefNum Registry Get.vi"("refnum name"="chasis") -> ("error out"=w220:errorcluster, "RobotDriveDevRef"=w221:T13)  [unwired: 9 in]
                n120 = call-poly <vilib>:"WPI_RobotDriveArcadeDrive.vi"("error in (no error)"=w220, "Y axis value"=-0.5 ("Motor Output"), "X axis value"=0.5 ("Motor Output"), "RobotDriveDevRef"=w221) -> ("error out"=w219:errorcluster, "RobotDriveDevRef"=w218:T13)  [unwired: 5 in, 1 out]
                n121 = call <vilib>:"WPI_RobotDriveDelayAndUpdateSafety.vi"("error in (no error)"=w219, "Delay (s)"=15.0, "RobotDriveDevRef"=w218) -> ()  [unwired: 7 in, 2 out]
              }
              frame #1 {
                n122 = call <vilib>:"WPI_RobotDriveRefNum Registry Get.vi"("refnum name"="chasis") -> ("error out"=w228:errorcluster, "RobotDriveDevRef"=w229:T13)  [unwired: 9 in]
                n123 = call-poly <vilib>:"WPI_RobotDriveArcadeDrive.vi"("error in (no error)"=w228, "Y axis value"=0.5 ("Motor Output"), "X axis value"=0.5 ("Motor Output"), "RobotDriveDevRef"=w229) -> ("error out"=w226:errorcluster, "RobotDriveDevRef"=w227:T13)  [unwired: 5 in, 1 out]
                n124 = call <vilib>:"WPI_RobotDriveDelayAndUpdateSafety.vi"("error in (no error)"=w226, "Delay (s)"=20.0, "RobotDriveDevRef"=w227) -> ()  [unwired: 7 in, 2 out]
              }
              frame #2 {
                w235 = 0.0 ("Motor Output")
                n125 = call <vilib>:"WPI_RobotDriveRefNum Registry Get.vi"("refnum name"="chasis") -> ("error out"=w233:errorcluster, "RobotDriveDevRef"=w234:T13)  [unwired: 9 in]
                n126 = call-poly <vilib>:"WPI_RobotDriveArcadeDrive.vi"("error in (no error)"=w233, "Y axis value"=w235, "X axis value"=w235, "RobotDriveDevRef"=w234) -> ()  [unwired: 5 in, 3 out]
              }
              frame #3 {
              }
            }
          }
          frame 4 {
            n127 = flat-sequence {
              tunnel: [5.0] -> w238
              frame #0 {
                n128 = call <vilib>:"WPI_MotorControlRefNum Registry Get.vi"("refnum name"="bomberos") -> ("error out"=w247:errorcluster, "MotorControlDevRef"=w246:T6)  [unwired: 9 in]
                n129 = call <vilib>:"WPI_MotorControlSetOutput.vi"("error in (no error)"=w247, "Output"=-0.5 ("Motor Output"), "MotorControlDevRef"=w246) -> ()  [unwired: 6 in, 3 out]
                n130 = Wait (ms)(milliseconds to wait=u32 20) -> ()  [unwired: 1 out]
                n131 = call <vilib>:"WPI_MotorControlRefNum Registry Get.vi"("refnum name"="polea") -> ("error out"=w243:errorcluster, "MotorControlDevRef"=w242:T6)  [unwired: 9 in]
                n132 = call <vilib>:"WPI_MotorControlSetOutput.vi"("error in (no error)"=w243, "Output"=0.5 ("Motor Output"), "MotorControlDevRef"=w242) -> ()  [unwired: 6 in, 3 out]
              }
              frame #1 {
                n133 = call <vilib>:"WPI_MotorControlRefNum Registry Get.vi"("refnum name"="polea") -> ("error out"=w254:errorcluster, "MotorControlDevRef"=w255:T6)  [unwired: 9 in]
                n134 = call <vilib>:"WPI_MotorControlRefNum Registry Get.vi"("refnum name"="bomberos") -> ("error out"=w252:errorcluster, "MotorControlDevRef"=w253:T6)  [unwired: 9 in]
                n135 = call <vilib>:"WPI_MotorControlSetOutput.vi"("error in (no error)"=w254, "Output"=0.0 ("Motor Output"), "MotorControlDevRef"=w255) -> ()  [unwired: 6 in, 3 out]
                n136 = call <vilib>:"WPI_MotorControlSetOutput.vi"("error in (no error)"=w252, "Output"=0.0 ("Motor Output"), "MotorControlDevRef"=w253) -> ()  [unwired: 6 in, 3 out]
              }
              frame #2 {
              }
            }
          }
          frame 5 {
            n137 = flat-sequence {
              tunnel: [6.0] -> w257
              frame #0 {
                n138 = call <vilib>:"WPI_SolenoidRefNum Registry Get.vi"("refnum name"="pickup") -> ("SolenoidDevRef"=w260:T11)  [unwired: 9 in, 1 out]
                n139 = call-poly <vilib>:"WPI_SolenoidSet.vi"("Value"=WPI_SolenoidValue."Reverse", "SolenoidDevRef"=w260) -> ()  [unwired: 8 in, 2 out]
              }
              frame #1 {
                n140 = Wait (ms)(milliseconds to wait=u32 200) -> ()  [unwired: 1 out]
              }
              frame #2 {
                n141 = call <vilib>:"WPI_SolenoidRefNum Registry Get.vi"("refnum name"="pickup") -> ("SolenoidDevRef"=w264:T11)  [unwired: 9 in, 1 out]
                n142 = call-poly <vilib>:"WPI_SolenoidSet.vi"("Value"=WPI_SolenoidValue."Forward", "SolenoidDevRef"=w264) -> ()  [unwired: 8 in, 2 out]
              }
              frame #3 {
              }
            }
          }
          frame 6 {
            n143 = flat-sequence {
              tunnel: [7.0] -> w266
              frame #0 {
                n144 = call <vilib>:"WPI_MotorControlRefNum Registry Get.vi"("refnum name"="polea") -> ("error out"=w275:errorcluster, "MotorControlDevRef"=w274:T6)  [unwired: 9 in]
                n145 = Wait (ms)(milliseconds to wait=u32 30) -> ()  [unwired: 1 out]
                n146 = call <vilib>:"WPI_MotorControlSetOutput.vi"("error in (no error)"=w275, "Output"=-0.5, "MotorControlDevRef"=w274) -> ()  [unwired: 6 in, 3 out]
                n147 = call <vilib>:"WPI_MotorControlRefNum Registry Get.vi"("refnum name"="bomberos") -> ("error out"=w271:errorcluster, "MotorControlDevRef"=w270:T6)  [unwired: 9 in]
                n148 = call <vilib>:"WPI_MotorControlSetOutput.vi"("error in (no error)"=w271, "Output"=-0.5, "MotorControlDevRef"=w270) -> ()  [unwired: 6 in, 3 out]
              }
              frame #1 {
                n149 = call <vilib>:"WPI_MotorControlRefNum Registry Get.vi"("refnum name"="polea") -> ("error out"=w282:errorcluster, "MotorControlDevRef"=w283:T6)  [unwired: 9 in]
                n150 = call <vilib>:"WPI_MotorControlRefNum Registry Get.vi"("refnum name"="bomberos") -> ("error out"=w278:errorcluster, "MotorControlDevRef"=w279:T6)  [unwired: 9 in]
                n151 = call <vilib>:"WPI_MotorControlSetOutput.vi"("error in (no error)"=w282, "Output"=0.0, "MotorControlDevRef"=w283) -> ()  [unwired: 6 in, 3 out]
                n152 = call <vilib>:"WPI_MotorControlSetOutput.vi"("error in (no error)"=w278, "Output"=0.0, "MotorControlDevRef"=w279) -> ()  [unwired: 6 in, 3 out]
              }
              frame #2 {
              }
            }
          }
          frame 7 {
            n153 = flat-sequence {
              tunnel: [8.0] -> w285
              frame #0 {
                n154 = call <vilib>:"WPI_RobotDriveRefNum Registry Get.vi"("refnum name"="chasis") -> ("error out"=w289:errorcluster, "RobotDriveDevRef"=w290:T13)  [unwired: 9 in]
                n155 = call-poly <vilib>:"WPI_RobotDriveArcadeDrive.vi"("error in (no error)"=w289, "Y axis value"=-0.5 ("Motor Output"), "X axis value"=0.5 ("Motor Output"), "RobotDriveDevRef"=w290) -> ("error out"=w287:errorcluster, "RobotDriveDevRef"=w288:T13)  [unwired: 5 in, 1 out]
                n156 = call <vilib>:"WPI_RobotDriveDelayAndUpdateSafety.vi"("error in (no error)"=w287, "Delay (s)"=29.0, "RobotDriveDevRef"=w288) -> ()  [unwired: 7 in, 2 out]
              }
              frame #1 {
                n157 = call <vilib>:"WPI_RobotDriveRefNum Registry Get.vi"("refnum name"="chasis") -> ("error out"=w298:errorcluster, "RobotDriveDevRef"=w299:T13)  [unwired: 9 in]
                n158 = call-poly <vilib>:"WPI_RobotDriveArcadeDrive.vi"("error in (no error)"=w298, "Y axis value"=0.5 ("Motor Output"), "X axis value"=0.5 ("Motor Output"), "RobotDriveDevRef"=w299) -> ("error out"=w296:errorcluster, "RobotDriveDevRef"=w295:T13)  [unwired: 5 in, 1 out]
                n159 = call <vilib>:"WPI_RobotDriveDelayAndUpdateSafety.vi"("error in (no error)"=w296, "Delay (s)"=29.0, "RobotDriveDevRef"=w295) -> ()  [unwired: 7 in, 2 out]
              }
              frame #2 {
                w302 = 0.0 ("Motor Output")
                n160 = call <vilib>:"WPI_RobotDriveRefNum Registry Get.vi"("refnum name"="chasis") -> ("error out"=w303:errorcluster, "RobotDriveDevRef"=w304:T13)  [unwired: 9 in]
                n161 = call-poly <vilib>:"WPI_RobotDriveArcadeDrive.vi"("error in (no error)"=w303, "Y axis value"=w302, "X axis value"=w302, "RobotDriveDevRef"=w304) -> ()  [unwired: 5 in, 3 out]
              }
              frame #3 {
              }
            }
          }
          frame 8 {
            n162 = flat-sequence {
              tunnel: [9.0] -> w308
              tunnel: [FALSE] -> w307
              frame #0 {
                n163 = call <vilib>:"WPI_SolenoidRefNum Registry Get.vi"("refnum name"="pickup") -> ("SolenoidDevRef"=w311:T11)  [unwired: 9 in, 1 out]
                n164 = call-poly <vilib>:"WPI_SolenoidSet.vi"("Value"=WPI_SolenoidValue."Reverse", "SolenoidDevRef"=w311) -> ()  [unwired: 8 in, 2 out]
                n165 = Wait (ms)(milliseconds to wait=u32 200) -> ()  [unwired: 1 out]
              }
              frame #1 {
                n166 = call <vilib>:"WPI_SolenoidRefNum Registry Get.vi"("refnum name"="pickup") -> ("SolenoidDevRef"=w315:T11)  [unwired: 9 in, 1 out]
                n167 = call-poly <vilib>:"WPI_SolenoidSet.vi"("Value"=WPI_SolenoidValue."Forward", "SolenoidDevRef"=w315) -> ()  [unwired: 8 in, 2 out]
              }
              frame #2 {
              }
            }
          }
        }
      }
    }
    frame "Caso 2" {
      n168 = while {
        shift-right: [w320] -> _
        shift-left: 1.0 -> [w321]
        stop <- w319 stop-if-true
        n169 = case shown="8" w321 {
          tunnel: [1.0 w323 w356 w365 w395 w428 w437 w470 w501] -> w320
          tunnel: [_ _ _ _ _ _ _ _ w500] -> w319
          frame 0, Default {
          }
          frame 1 {
            n170 = flat-sequence {
              tunnel: [2.0] -> w323
              frame #0 {
                n171 = call <vilib>:"WPI_MotorControlRefNum Registry Get.vi"("refnum name"="bomberos") -> ("error out"=w324:errorcluster, "MotorControlDevRef"=w325:T6)  [unwired: 9 in]
                n172 = call <vilib>:"WPI_MotorControlRefNum Registry Get.vi"("refnum name"="polea") -> ("error out"=w328:errorcluster, "MotorControlDevRef"=w329:T6)  [unwired: 9 in]
                n173 = call <vilib>:"Spark MAX Set Sensor Position.vi"("error in"=w324, "Position"=0.0, "MotorControlDeviceRef"=w325) -> ()  [unwired: 7 in, 2 out]
                n174 = call <vilib>:"Spark MAX Set Sensor Position.vi"("error in"=w328, "Position"=0.0, "MotorControlDeviceRef"=w329) -> ()  [unwired: 7 in, 2 out]
              }
              frame #1 {
                n175 = while {
                  stop <- w335 stop-if-true
                  n176 = call <vilib>:"WPI_MotorControlRefNum Registry Get.vi"("refnum name"="polea") -> ("error out"=w345:errorcluster, "MotorControlDevRef"=w346:T6)  [unwired: 9 in]
                  n177 = global read "Robot Global Data.vi" "bomberos"() -> (w334:dbl)
                  n178 = global read "Robot Global Data.vi" "vpolea"() -> (w342:dbl)
                  n179 = call <vilib>:"WPI_MotorControlSetOutput.vi"("error in (no error)"=w345, "Output"=-0.5 ("Motor Output"), "MotorControlDevRef"=w346) -> ()  [unwired: 6 in, 3 out]
                  n180 = Greater Or Equal?(x=w334, y=15.0) -> (x >= y?=w332:bool)
                  n181 = Greater Or Equal?(x=w342, y=15.0) -> (x >= y?=w336:bool)
                  n182 = call <vilib>:"WPI_MotorControlRefNum Registry Get.vi"("refnum name"="bomberos") -> ("error out"=w340:errorcluster, "MotorControlDevRef"=w339:T6)  [unwired: 9 in]
                  n183 = And(x=w336, y=w332) -> (x .and. y?=w335:bool)
                  n184 = call <vilib>:"WPI_MotorControlSetOutput.vi"("error in (no error)"=w340, "Output"=0.5 ("Motor Output"), "MotorControlDevRef"=w339) -> ()  [unwired: 6 in, 3 out]
                }
              }
              frame #2 {
                n185 = call <vilib>:"WPI_MotorControlRefNum Registry Get.vi"("refnum name"="bomberos") -> ("error out"=w349:errorcluster, "MotorControlDevRef"=w350:T6)  [unwired: 9 in]
                n186 = call <vilib>:"WPI_MotorControlRefNum Registry Get.vi"("refnum name"="polea") -> ("error out"=w353:errorcluster, "MotorControlDevRef"=w354:T6)  [unwired: 9 in]
                n187 = call <vilib>:"WPI_MotorControlSetOutput.vi"("error in (no error)"=w349, "Output"=0.0 ("Motor Output"), "MotorControlDevRef"=w350) -> ()  [unwired: 6 in, 3 out]
                n188 = call <vilib>:"WPI_MotorControlSetOutput.vi"("error in (no error)"=w353, "Output"=0.0 ("Motor Output"), "MotorControlDevRef"=w354) -> ()  [unwired: 6 in, 3 out]
              }
              frame #3 {
              }
            }
          }
          frame 2 {
            n189 = flat-sequence {
              tunnel: [3.0] -> w356
              frame #0 {
                n190 = call <vilib>:"WPI_SolenoidRefNum Registry Get.vi"("refnum name"="pickup") -> ("SolenoidDevRef"=w359:T11)  [unwired: 9 in, 1 out]
                n191 = call-poly <vilib>:"WPI_SolenoidSet.vi"("Value"=WPI_SolenoidValue."Reverse", "SolenoidDevRef"=w359) -> ()  [unwired: 8 in, 2 out]
              }
              frame #1 {
                n192 = Wait (ms)(milliseconds to wait=u32 200) -> ()  [unwired: 1 out]
              }
              frame #2 {
                n193 = call <vilib>:"WPI_SolenoidRefNum Registry Get.vi"("refnum name"="pickup") -> ("SolenoidDevRef"=w363:T11)  [unwired: 9 in, 1 out]
                n194 = call-poly <vilib>:"WPI_SolenoidSet.vi"("Value"=WPI_SolenoidValue."Forward", "SolenoidDevRef"=w363) -> ()  [unwired: 8 in, 2 out]
              }
              frame #3 {
              }
            }
          }
          frame 3 {
            n195 = flat-sequence {
              tunnel: [4.0] -> w365
              frame #0 {
                n196 = call <vilib>:"WPI_MotorControlRefNum Registry Get.vi"("refnum name"="llantas") -> ("error out"=w366:errorcluster, "MotorControlDevRef"=w367:T6)  [unwired: 9 in]
                n197 = call <vilib>:"Spark MAX Set Sensor Position.vi"("error in"=w366, "Position"=0.0, "MotorControlDeviceRef"=w367) -> ()  [unwired: 7 in, 2 out]
              }
              frame #1 {
                n198 = while {
                  stop <- w374 stop-if-true
                  # "da vuelta"
                  n199 = global read "Robot Global Data.vi" "ruedas"() -> (w376:dbl)
                  n200 = call <vilib>:"WPI_RobotDriveRefNum Registry Get.vi"("refnum name"="chasis") -> ("error out"=w370:errorcluster, "RobotDriveDevRef"=w371:T13)  [unwired: 9 in]
                  n201 = Greater Or Equal?(x=w376, y=40.0) -> (x >= y?=w374:bool)
                  n202 = call-poly <vilib>:"WPI_RobotDriveArcadeDrive.vi"("error in (no error)"=w370, "Y axis value"=-0.5 ("Motor Output"), "X axis value"=0.5 ("Motor Output"), "RobotDriveDevRef"=w371) -> ()  [unwired: 5 in, 3 out]
                }
              }
              frame #2 {
                n203 = call <vilib>:"WPI_MotorControlRefNum Registry Get.vi"("refnum name"="llantas") -> ("error out"=w378:errorcluster, "MotorControlDevRef"=w379:T6)  [unwired: 9 in]
                n204 = call <vilib>:"Spark MAX Set Sensor Position.vi"("error in"=w378, "Position"=0.0, "MotorControlDeviceRef"=w379) -> ()  [unwired: 7 in, 2 out]
              }
              frame #3 {
                n205 = while {
                  stop <- w386 stop-if-true
                  # "avanza"
                  n206 = global read "Robot Global Data.vi" "ruedas"() -> (w388:dbl)
                  n207 = call <vilib>:"WPI_RobotDriveRefNum Registry Get.vi"("refnum name"="chasis") -> ("error out"=w382:errorcluster, "RobotDriveDevRef"=w383:T13)  [unwired: 9 in]
                  n208 = Greater Or Equal?(x=w388, y=50.0) -> (x >= y?=w386:bool)
                  n209 = call-poly <vilib>:"WPI_RobotDriveArcadeDrive.vi"("error in (no error)"=w382, "Y axis value"=0.5 ("Motor Output"), "X axis value"=0.5 ("Motor Output"), "RobotDriveDevRef"=w383) -> ()  [unwired: 5 in, 3 out]
                }
              }
              frame #4 {
                w392 = 0.0 ("Motor Output")
                n210 = call <vilib>:"WPI_RobotDriveRefNum Registry Get.vi"("refnum name"="chasis") -> ("error out"=w390:errorcluster, "RobotDriveDevRef"=w391:T13)  [unwired: 9 in]
                n211 = call-poly <vilib>:"WPI_RobotDriveArcadeDrive.vi"("error in (no error)"=w390, "Y axis value"=w392, "X axis value"=w392, "RobotDriveDevRef"=w391) -> ()  [unwired: 5 in, 3 out]
              }
              frame #5 {
              }
            }
          }
          frame 4 {
            n212 = flat-sequence {
              tunnel: [5.0] -> w395
              frame #0 {
                n213 = call <vilib>:"WPI_MotorControlRefNum Registry Get.vi"("refnum name"="polea") -> ("error out"=w396:errorcluster, "MotorControlDevRef"=w397:T6)  [unwired: 9 in]
                n214 = call <vilib>:"Spark MAX Set Sensor Position.vi"("error in"=w396, "Position"=0.0, "MotorControlDeviceRef"=w397) -> ()  [unwired: 7 in, 2 out]
                n215 = call <vilib>:"WPI_MotorControlRefNum Registry Get.vi"("refnum name"="bomberos") -> ("error out"=w400:errorcluster, "MotorControlDevRef"=w401:T6)  [unwired: 9 in]
                n216 = call <vilib>:"Spark MAX Set Sensor Position.vi"("error in"=w400, "Position"=0.0, "MotorControlDeviceRef"=w401) -> ()  [unwired: 7 in, 2 out]
              }
              frame #1 {
                n217 = while {
                  stop <- w408 stop-if-true
                  n218 = global read "Robot Global Data.vi" "bomberos"() -> (w410:dbl)
                  n219 = call <vilib>:"WPI_MotorControlRefNum Registry Get.vi"("refnum name"="bomberos") -> ("error out"=w418:errorcluster, "MotorControlDevRef"=w417:T6)  [unwired: 9 in]
                  n220 = global read "Robot Global Data.vi" "vpolea"() -> (w406:dbl)
                  n221 = call <vilib>:"WPI_MotorControlSetOutput.vi"("error in (no error)"=w418, "Output"=-0.5 ("Motor Output"), "MotorControlDevRef"=w417) -> ()  [unwired: 6 in, 3 out]
                  n222 = Greater Or Equal?(x=w410, y=20.0) -> (x >= y?=w409:bool)
                  n223 = Greater Or Equal?(x=w406, y=20.0) -> (x >= y?=w404:bool)
                  n224 = call <vilib>:"WPI_MotorControlRefNum Registry Get.vi"("refnum name"="polea") -> ("error out"=w414:errorcluster, "MotorControlDevRef"=w413:T6)  [unwired: 9 in]
                  n225 = And(x=w409, y=w404) -> (x .and. y?=w408:bool)
                  n226 = call <vilib>:"WPI_MotorControlSetOutput.vi"("error in (no error)"=w414, "Output"=0.5 ("Motor Output"), "MotorControlDevRef"=w413) -> ()  [unwired: 6 in, 3 out]
                }
              }
              frame #2 {
                n227 = call <vilib>:"WPI_MotorControlRefNum Registry Get.vi"("refnum name"="polea") -> ("error out"=w425:errorcluster, "MotorControlDevRef"=w426:T6)  [unwired: 9 in]
                n228 = call <vilib>:"WPI_MotorControlRefNum Registry Get.vi"("refnum name"="bomberos") -> ("error out"=w423:errorcluster, "MotorControlDevRef"=w424:T6)  [unwired: 9 in]
                n229 = call <vilib>:"WPI_MotorControlSetOutput.vi"("error in (no error)"=w425, "Output"=0.0 ("Motor Output"), "MotorControlDevRef"=w426) -> ()  [unwired: 6 in, 3 out]
                n230 = call <vilib>:"WPI_MotorControlSetOutput.vi"("error in (no error)"=w423, "Output"=0.0 ("Motor Output"), "MotorControlDevRef"=w424) -> ()  [unwired: 6 in, 3 out]
              }
              frame #3 {
              }
            }
          }
          frame 5 {
            n231 = flat-sequence {
              tunnel: [6.0] -> w428
              frame #0 {
                n232 = call <vilib>:"WPI_SolenoidRefNum Registry Get.vi"("refnum name"="pickup") -> ("SolenoidDevRef"=w431:T11)  [unwired: 9 in, 1 out]
                n233 = call-poly <vilib>:"WPI_SolenoidSet.vi"("Value"=WPI_SolenoidValue."Reverse", "SolenoidDevRef"=w431) -> ()  [unwired: 8 in, 2 out]
              }
              frame #1 {
                n234 = Wait (ms)(milliseconds to wait=u32 200) -> ()  [unwired: 1 out]
              }
              frame #2 {
                n235 = call <vilib>:"WPI_SolenoidRefNum Registry Get.vi"("refnum name"="pickup") -> ("SolenoidDevRef"=w435:T11)  [unwired: 9 in, 1 out]
                n236 = call-poly <vilib>:"WPI_SolenoidSet.vi"("Value"=WPI_SolenoidValue."Forward", "SolenoidDevRef"=w435) -> ()  [unwired: 8 in, 2 out]
              }
              frame #3 {
              }
            }
          }
          frame 6 {
            n237 = flat-sequence {
              tunnel: [7.0] -> w437
              frame #0 {
                n238 = call <vilib>:"WPI_MotorControlRefNum Registry Get.vi"("refnum name"="bomberos") -> ("error out"=w442:errorcluster, "MotorControlDevRef"=w443:T6)  [unwired: 9 in]
                n239 = call <vilib>:"WPI_MotorControlRefNum Registry Get.vi"("refnum name"="polea") -> ("error out"=w438:errorcluster, "MotorControlDevRef"=w439:T6)  [unwired: 9 in]
                n240 = call <vilib>:"Spark MAX Set Sensor Position.vi"("error in"=w442, "Position"=0.0, "MotorControlDeviceRef"=w443) -> ()  [unwired: 7 in, 2 out]
                n241 = call <vilib>:"Spark MAX Set Sensor Position.vi"("error in"=w438, "Position"=0.0, "MotorControlDeviceRef"=w439) -> ()  [unwired: 7 in, 2 out]
              }
              frame #1 {
                n242 = while {
                  stop <- w449 stop-if-true
                  n243 = global read "Robot Global Data.vi" "bomberos"() -> (w448:dbl)
                  n244 = global read "Robot Global Data.vi" "vpolea"() -> (w456:dbl)
                  n245 = call <vilib>:"WPI_MotorControlRefNum Registry Get.vi"("refnum name"="polea") -> ("error out"=w460:errorcluster, "MotorControlDevRef"=w459:T6)  [unwired: 9 in]
                  n246 = Equal?(x=w448, y=15.0) -> (x = y?=w446:bool)
                  n247 = call <vilib>:"WPI_MotorControlSetOutput.vi"("error in (no error)"=w460, "Output"=-0.5, "MotorControlDevRef"=w459) -> ()  [unwired: 6 in, 3 out]
                  n248 = Equal?(x=w456, y=15.0) -> (x = y?=w450:bool)
                  n249 = call <vilib>:"WPI_MotorControlRefNum Registry Get.vi"("refnum name"="bomberos") -> ("error out"=w454:errorcluster, "MotorControlDevRef"=w453:T6)  [unwired: 9 in]
                  n250 = And(x=w450, y=w446) -> (x .and. y?=w449:bool)
                  n251 = call <vilib>:"WPI_MotorControlSetOutput.vi"("error in (no error)"=w454, "Output"=-0.5, "MotorControlDevRef"=w453) -> ()  [unwired: 6 in, 3 out]
                }
              }
              frame #2 {
                n252 = call <vilib>:"WPI_MotorControlRefNum Registry Get.vi"("refnum name"="polea") -> ("error out"=w467:errorcluster, "MotorControlDevRef"=w468:T6)  [unwired: 9 in]
                n253 = call <vilib>:"WPI_MotorControlRefNum Registry Get.vi"("refnum name"="bomberos") -> ("error out"=w463:errorcluster, "MotorControlDevRef"=w464:T6)  [unwired: 9 in]
                n254 = call <vilib>:"WPI_MotorControlSetOutput.vi"("error in (no error)"=w467, "Output"=0.0, "MotorControlDevRef"=w468) -> ()  [unwired: 6 in, 3 out]
                n255 = call <vilib>:"WPI_MotorControlSetOutput.vi"("error in (no error)"=w463, "Output"=0.0, "MotorControlDevRef"=w464) -> ()  [unwired: 6 in, 3 out]
              }
              frame #3 {
              }
            }
          }
          frame 7 {
            n256 = flat-sequence {
              tunnel: [8.0] -> w470
              frame #0 {
                n257 = call <vilib>:"WPI_MotorControlRefNum Registry Get.vi"("refnum name"="llanta") -> ("error out"=w471:errorcluster, "MotorControlDevRef"=w472:T6)  [unwired: 9 in]
                n258 = call <vilib>:"Spark MAX Set Sensor Position.vi"("error in"=w471, "Position"=0.0, "MotorControlDeviceRef"=w472) -> ()  [unwired: 7 in, 2 out]
              }
              frame #1 {
                n259 = while {
                  stop <- w479 stop-if-true
                  # "da vuelta"
                  n260 = global read "Robot Global Data.vi" "ruedas"() -> (w481:dbl)
                  n261 = call <vilib>:"WPI_RobotDriveRefNum Registry Get.vi"("refnum name"="chasis") -> ("error out"=w475:errorcluster, "RobotDriveDevRef"=w476:T13)  [unwired: 9 in]
                  n262 = Equal?(x=w481, y=40.0) -> (x = y?=w479:bool)
                  n263 = call-poly <vilib>:"WPI_RobotDriveArcadeDrive.vi"("error in (no error)"=w475, "Y axis value"=-0.5 ("Motor Output"), "X axis value"=0.5 ("Motor Output"), "RobotDriveDevRef"=w476) -> ()  [unwired: 5 in, 3 out]
                }
              }
              frame #2 {
                n264 = call <vilib>:"WPI_MotorControlRefNum Registry Get.vi"("refnum name"="llanta") -> ("error out"=w483:errorcluster, "MotorControlDevRef"=w484:T6)  [unwired: 9 in]
                n265 = call <vilib>:"Spark MAX Set Sensor Position.vi"("error in"=w483, "Position"=0.0, "MotorControlDeviceRef"=w484) -> ()  [unwired: 7 in, 2 out]
              }
              frame #3 {
                n266 = while {
                  stop <- w491 stop-if-true
                  # "avanza"
                  n267 = global read "Robot Global Data.vi" "ruedas"() -> (w493:dbl)
                  n268 = call <vilib>:"WPI_RobotDriveRefNum Registry Get.vi"("refnum name"="chasis") -> ("error out"=w487:errorcluster, "RobotDriveDevRef"=w488:T13)  [unwired: 9 in]
                  n269 = Equal?(x=w493, y=50.0) -> (x = y?=w491:bool)
                  n270 = call-poly <vilib>:"WPI_RobotDriveArcadeDrive.vi"("error in (no error)"=w487, "Y axis value"=0.5 ("Motor Output"), "X axis value"=0.5 ("Motor Output"), "RobotDriveDevRef"=w488) -> ()  [unwired: 5 in, 3 out]
                }
              }
              frame #4 {
                w495 = 0.0 ("Motor Output")
                n271 = call <vilib>:"WPI_RobotDriveRefNum Registry Get.vi"("refnum name"="chasis") -> ("error out"=w496:errorcluster, "RobotDriveDevRef"=w497:T13)  [unwired: 9 in]
                n272 = call-poly <vilib>:"WPI_RobotDriveArcadeDrive.vi"("error in (no error)"=w496, "Y axis value"=w495, "X axis value"=w495, "RobotDriveDevRef"=w497) -> ()  [unwired: 5 in, 3 out]
              }
              frame #5 {
              }
            }
          }
          frame 8 {
            n273 = flat-sequence {
              tunnel: [9.0] -> w501
              tunnel: [FALSE] -> w500
              frame #0 {
                n274 = call <vilib>:"WPI_SolenoidRefNum Registry Get.vi"("refnum name"="pickup") -> ("SolenoidDevRef"=w504:T11)  [unwired: 9 in, 1 out]
                n275 = call-poly <vilib>:"WPI_SolenoidSet.vi"("Value"=WPI_SolenoidValue."Reverse", "SolenoidDevRef"=w504) -> ()  [unwired: 8 in, 2 out]
              }
              frame #1 {
                n276 = Wait (ms)(milliseconds to wait=u32 200) -> ()  [unwired: 1 out]
              }
              frame #2 {
                n277 = call <vilib>:"WPI_SolenoidRefNum Registry Get.vi"("refnum name"="pickup") -> ("SolenoidDevRef"=w508:T11)  [unwired: 9 in, 1 out]
                n278 = call-poly <vilib>:"WPI_SolenoidSet.vi"("Value"=WPI_SolenoidValue."Forward", "SolenoidDevRef"=w508) -> ()  [unwired: 8 in, 2 out]
              }
              frame #3 {
              }
            }
          }
        }
      }
    }
  }
